vi "BRig_RT__Case_Exp__State_initTrial__LC_ENL__v10.vi"(6 "input_arrTrig":bool[](array[boolean]), 8 "input_dataTrial":u16[][](array[numeric]), 9 "input_dataExp":u16[](array[numeric]), 10 "input_dataLC":u16[](array[numeric]), 11 "input_dataCurrent":u16[](array[numeric])) -> (0 "output_dataTrial":u16[][](array[numeric]), 3 "output_dataCurrent":u16[](array[numeric]), 4 "output_arrTrig":bool[](array[boolean]))   [LabVIEW 2014]
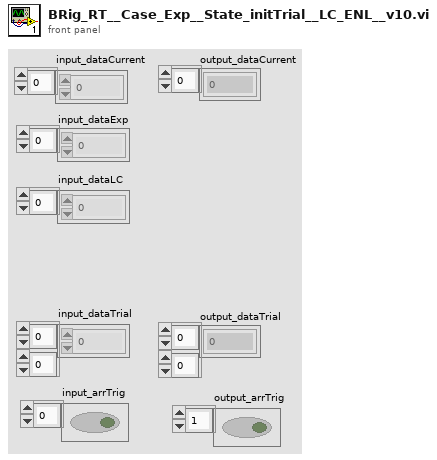
[diagram p1: front panel]
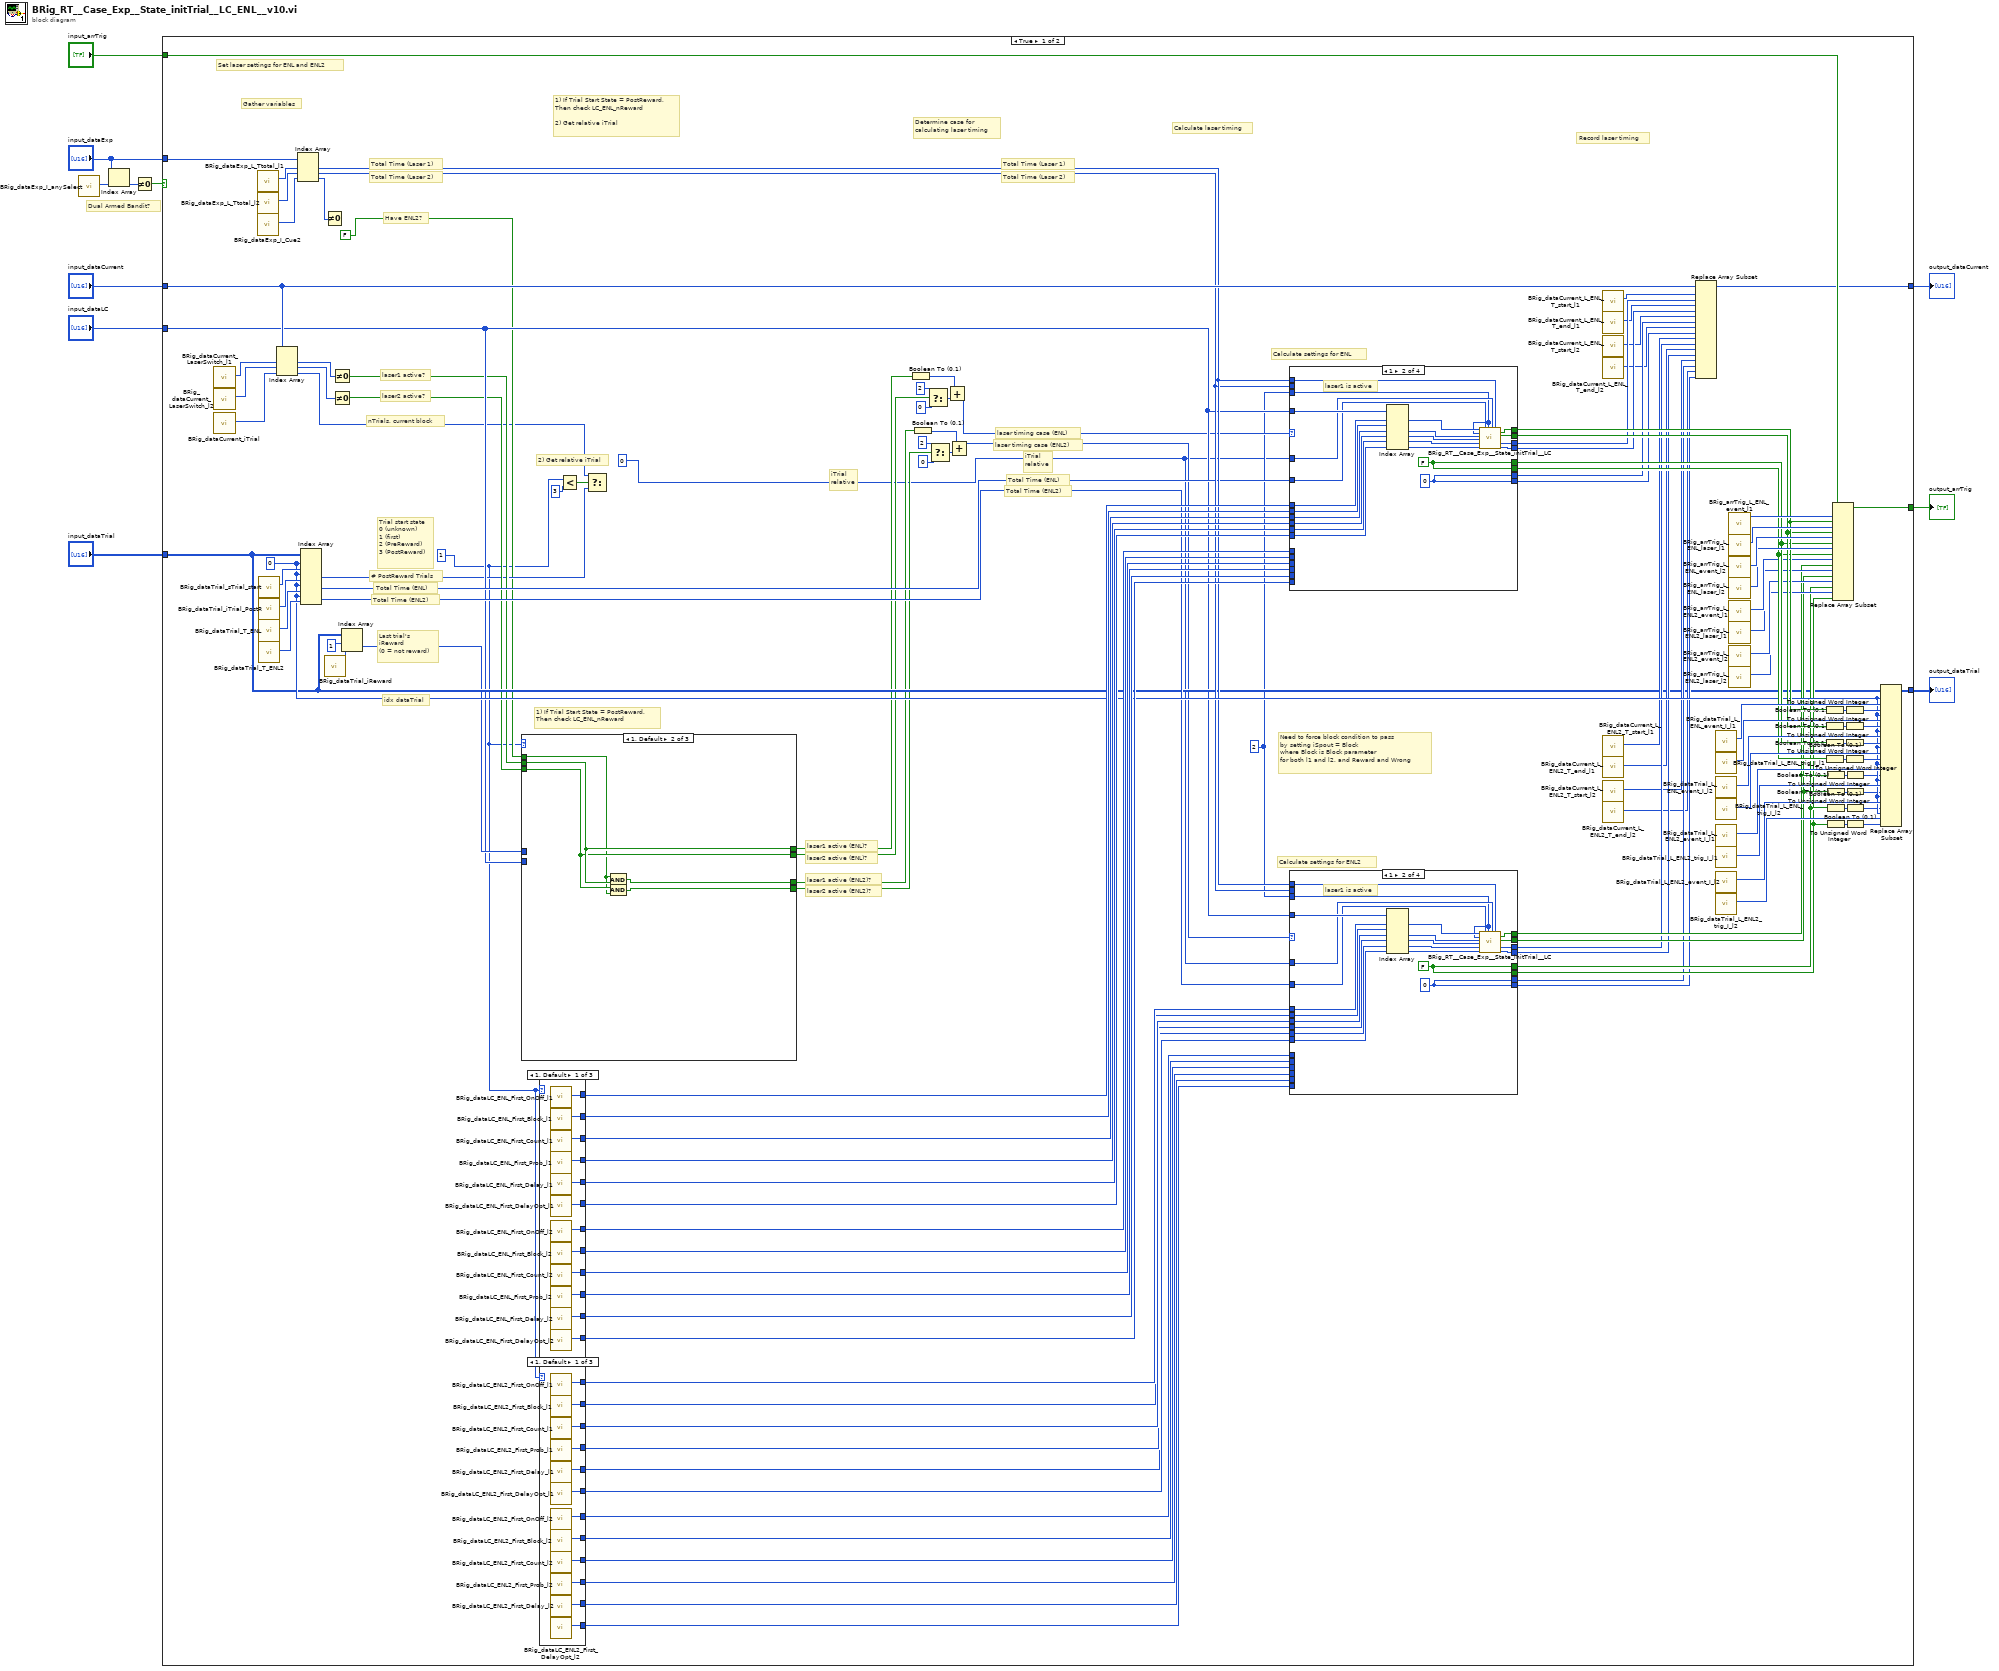
[diagram p0: block diagram]
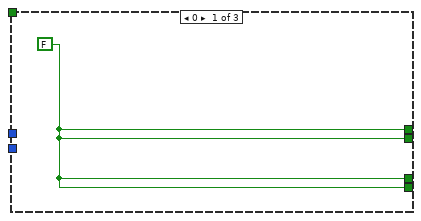
[diagram p2: hidden frame]
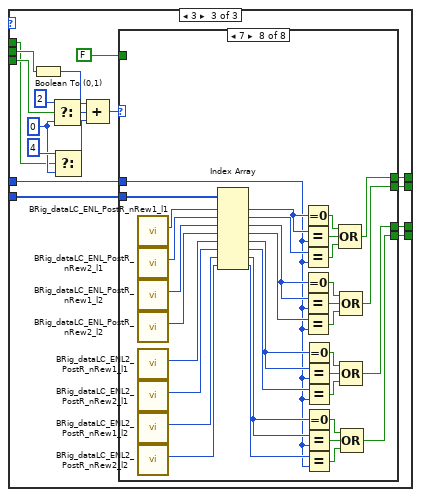
[diagram p3: hidden frame]
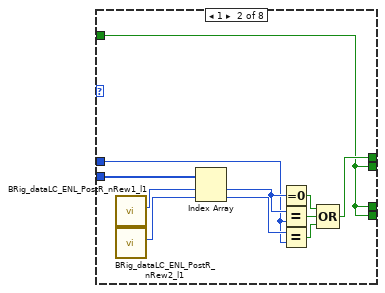
[diagram p5: hidden frame]
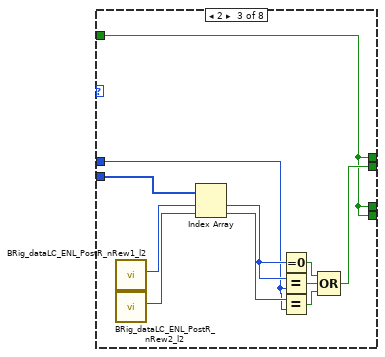
[diagram p6: hidden frame]
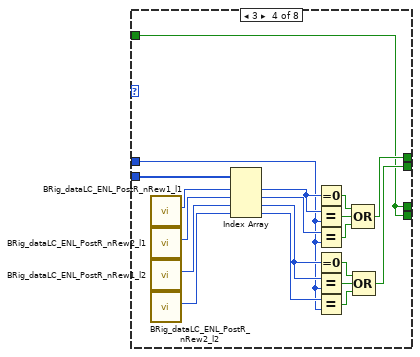
[diagram p7: hidden frame]
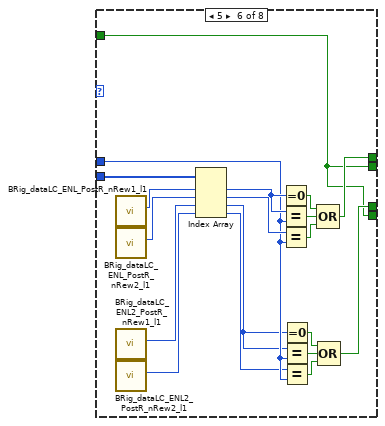
[diagram p9: hidden frame]
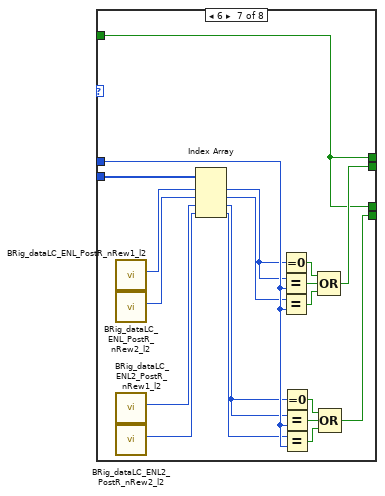
[diagram p10: hidden frame]
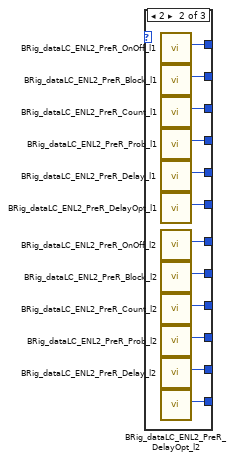
[diagram p11: hidden frame]
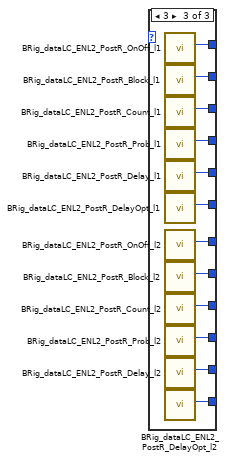
[diagram p12: hidden frame]
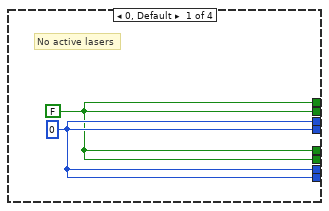
[diagram p13: hidden frame]
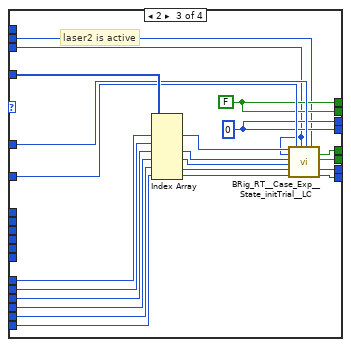
[diagram p14: hidden frame]
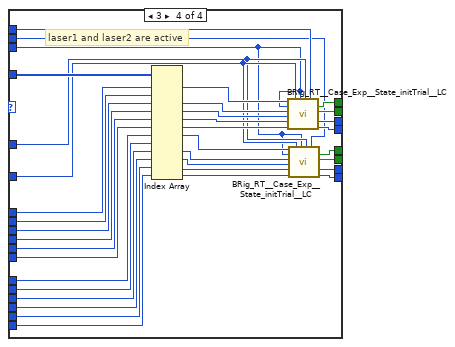
[diagram p15: hidden frame]
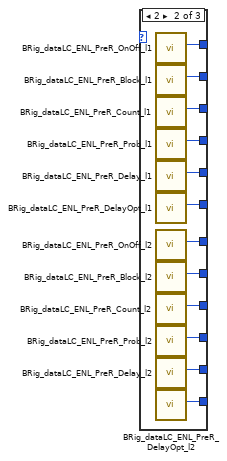
[diagram p16: hidden frame]
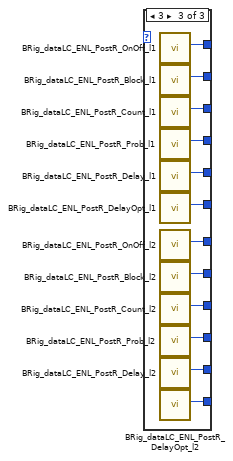
[diagram p17: hidden frame]
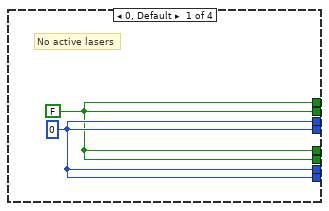
[diagram p18: hidden frame]
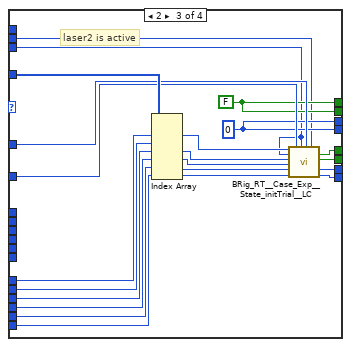
[diagram p19: hidden frame]
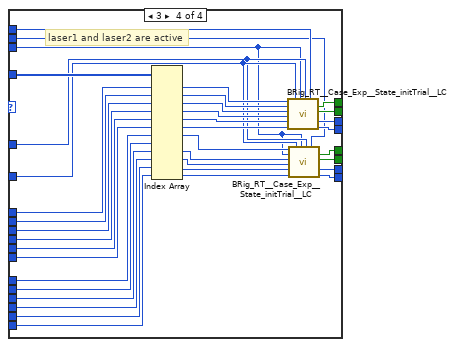
[diagram p20: hidden frame]
diagram:
  # "Dual Armed Bandit?"
  n1 = call "BRig_dataExp_I_anySelect.vi"() -> ("output_I_anySelect"=w4:i32)  [unwired: 11 in]
  n2 = Index Array(array="input_dataExp", index=w4) -> (element=w3:u16)
  n3 = Not Equal To 0?(x=w3) -> (x != 0?=w1:bool)
  n4 = case shown="True" w1 {
    tunnel: "input_arrTrig" -> [w135 w643]
    tunnel: [w134 w642] -> w10
    tunnel: [w113 w621] -> w9
    tunnel: "input_dataCurrent" -> [w112 w620]
    tunnel: [w111 w619] -> w7
    tunnel: "input_dataExp" -> [w88 w596]
    tunnel: "input_dataTrial" -> [w34 w541]
    tunnel: "input_dataLC" -> [w32 w539]
    frame True {
      w12 = u16 1
      w13 = u16 0
      w15 = u16 2 ("input_sState_start")
      w72 = 0
      # "Need to force block condition to pass\nby setting iSpout = Block\nwhere Block is Block parameter\nfor both l1 and l2, and Reward and Wrong"
      # "Record laser timing"
      # "Calculate laser timing"
      # "Total Time (ENL2)"
      # "Total Time (ENL)"
      # "iTrial\nrelative"
      # "Total Time (Laser 2)"
      # "Total Time (Laser 1)"
      # "laser timing case (ENL2)"
      # "Determine case for\ncalculating laser timing"
      # "2) Get relative iTrial"
      # "1) If Trial Start State = PostReward,\nThen check LC_ENL_nReward"
      # "laser2 active (ENL2)?"
      # "laser1 active (ENL2)?"
      # "laser2 active (ENL)?"
      # "laser1 active (ENL)?"
      # "1) If Trial Start State = PostReward,\nThen check LC_ENL_nReward\n\n2) Get relative iTrial"
      # "Gather variables"
      # "Last trial's\niReward\n(0 = not reward)"
      # "nTrials, current block"
      # "idx dataTrial"
      # "Total Time (ENL2)"
      # "Total Time (ENL)"
      # "# PostReward Trials"
      # "Have ENL2?"
      # "Total Time (Laser 2)"
      # "Total Time (Laser 1)"
      # "Calculate settings for ENL2"
      # "Calculate settings for ENL"
      # "Set laser settings for ENL and ENL2"
      # "iTrial\nrelative"
      # "laser timing case (ENL)"
      # "Trial start state\n0 (unknown)\n1 (first)\n2 (PreReward)\n3 (PostReward)"
      # "laser2 active?"
      # "laser1 active?"
      n5 = call "BRig_dataCurrent_LaserSwitch_l1.vi"() -> ("output_LaserSwitch_l1"=w144:i32)  [unwired: 11 in]
      n6 = call "BRig_dataCurrent_LaserSwitch_l2.vi"() -> ("output_LaserSwitch_l2"=w143:i32)  [unwired: 11 in]
      n7 = call "BRig_dataCurrent_iTrial.vi"() -> ("output_iTrial"=w85:i32)  [unwired: 11 in]
      n8 = call "BRig_dataExp_L_Ttotal_l1.vi"() -> ("output_L_Ttotal_l1"=w89:i32)  [unwired: 11 in]
      n9 = call "BRig_dataExp_L_Ttotal_l2.vi"() -> ("output_L_Ttotal_l2"=w90:i32)  [unwired: 11 in]
      n10 = call "BRig_dataExp_I_Cue2.vi"() -> ("output_I_Cue2"=w40:i32)  [unwired: 11 in]
      n11 = call "BRig_dataTrial_sTrial_start.vi"() -> ("output_sTrial_start"=w140:i32)  [unwired: 11 in]
      n12 = call "BRig_dataTrial_iTrial_PostR.vi"() -> ("output_iTrial_PostR"=w86:i32)  [unwired: 11 in]
      n13 = call "BRig_dataTrial_T_ENL.vi"() -> ("output_T_ENL"=w87:i32)  [unwired: 11 in]
      n14 = call "BRig_dataTrial_T_ENL2.vi"() -> ("output_T_ENL2"=w84:i32)  [unwired: 11 in]
      n15 = Index Array(array=w112, index #1=w144, index #2=w143, index #3=w85) -> (element #1=w142:u16, element #2=w141:u16, element #3=w14:u16)
      n16 = Index Array(array=w88, index #1=w89, index #2=w90, index #3=w40) -> (element #1=w66:u16, element #2=w65:u16, element #3=w39:u16)
      n17 = Index Array(array=w34, index (row) #1=w72, index (col) #1=w140, index (row) #2=w72, index (col) #2=w86, index (row) #3=w72, index (col) #3=w87, index (row) #4=w72, index (col) #4=w84) -> (element #2=w27:u16, element #3=w38:u16, element #4=w37:u16)  [unwired: 1 out]
      n18 = Not Equal To 0?(x=w39) -> ()  [unwired: 1 out]
      n19 = call "BRig_dataTrial_iReward.vi"() -> ("output_iReward"=w35:i32)  [unwired: 11 in]
      n20 = Not Equal To 0?(x=w142) -> (x != 0?=w30:bool)
      n21 = Not Equal To 0?(x=w141) -> (x != 0?=w31:bool)
      n22 = Index Array(array=w34, index (row)=1 ("disabled index (row)"), index (col)=w35) -> (element=w33:u16)
      n23 = case shown="1, Default" w12 {
        tunnel: w33 -> [_ _ w159]
        tunnel: w32 -> [_ _ w160]
        tunnel: w31 -> [_ w149 w152]
        tunnel: w30 -> [_ w150 w153]
        tunnel: FALSE -> [_ w148 w151]
        tunnel: [w145 w150 w158] -> w26
        tunnel: [w145 w149 w157] -> w25
        tunnel: [w145 w147 w156] -> w20
        tunnel: [w145 w146 w155] -> w19
        frame 0 {
          w145 = FALSE
        }
        frame 1, Default {
          n24 = And(x=w148, y=w150) -> (x .and. y?=w147:bool)
          n25 = And(x=w149, y=w148) -> (x .and. y?=w146:bool)
        }
        frame 3 {
          w165 = i16 0 ("f")
          n26 = Boolean To (0,1)(Boolean=w153) -> (0, 1=w163:i16)
          n27 = Select(t=i16 2, s=w152, f=w165) -> (s? t:f=w164:i16)
          n28 = Select(t=i16 4, s=w151, f=w165) -> (s? t:f=w162:i16)
          n29 = Compound Arithmetic op=ADD(w163, w164, w162) -> (w161:i16)
          n30 = case shown="7" w161 {
            tunnel: w160 -> [_ w172 w183 w195 _ w222 w245 w268]
            tunnel: w159 -> [_ w171 w182 w194 _ w218 w241 w253]
            tunnel: [w168 w170 w180 w193 w210 w217 w238 w252] -> w158
            tunnel: [w168 w169 w181 w192 w210 w215 w240 w251] -> w157
            tunnel: [w168 w169 w180 w191 w210 w216 w238 w250] -> w156
            tunnel: [w168 w169 w180 w191 w210 w215 w239 w249] -> w155
            tunnel: FALSE -> [w168 w169 w180 w191 w210 w215 w238 _]
            frame 0, Default {
            }
            frame 1 {
              n31 = call "BRig_dataLC_ENL_PostR_nRew1_l1.vi"() -> ("output_ENL_PostR_nRew1_l1"=w179:i32)  [unwired: 11 in]
              n32 = call "BRig_dataLC_ENL_PostR_nRew2_l1.vi"() -> ("output_ENL_PostR_nRew2_l1"=w178:i32)  [unwired: 11 in]
              n33 = Index Array(array=w172, index #1=w179, index #2=w178) -> (element #1=w174:u16, element #2=w173:u16)
              n34 = Equal To 0?(x=w174) -> (x = 0?=w175:bool)
              n35 = Equal?(x=w174, y=w171) -> (x = y?=w176:bool)
              n36 = Equal?(x=w173, y=w171) -> (x = y?=w177:bool)
              n37 = Compound Arithmetic op=OR(w175, w176, w177) -> (w170:bool)
            }
            frame 2 {
              n38 = call "BRig_dataLC_ENL_PostR_nRew1_l2.vi"() -> ("output_ENL_PostR_nRew1_l2"=w190:i32)  [unwired: 11 in]
              n39 = call "BRig_dataLC_ENL_PostR_nRew2_l2.vi"() -> ("output_ENL_PostR_nRew2_l2"=w189:i32)  [unwired: 11 in]
              n40 = Index Array(array=w183, index #1=w190, index #2=w189) -> (element #1=w184:u16, element #2=w185:u16)
              n41 = Equal To 0?(x=w184) -> (x = 0?=w187:bool)
              n42 = Equal?(x=w184, y=w182) -> (x = y?=w186:bool)
              n43 = Equal?(x=w185, y=w182) -> (x = y?=w188:bool)
              n44 = Compound Arithmetic op=OR(w187, w186, w188) -> (w181:bool)
            }
            frame 3 {
              n45 = call "BRig_dataLC_ENL_PostR_nRew1_l1.vi"() -> ("output_ENL_PostR_nRew1_l1"=w209:i32)  [unwired: 11 in]
              n46 = call "BRig_dataLC_ENL_PostR_nRew2_l1.vi"() -> ("output_ENL_PostR_nRew2_l1"=w208:i32)  [unwired: 11 in]
              n47 = call "BRig_dataLC_ENL_PostR_nRew1_l2.vi"() -> ("output_ENL_PostR_nRew1_l2"=w207:i32)  [unwired: 11 in]
              n48 = call "BRig_dataLC_ENL_PostR_nRew2_l2.vi"() -> ("output_ENL_PostR_nRew2_l2"=w206:i32)  [unwired: 11 in]
              n49 = Index Array(array=w195, index #1=w209, index #2=w208, index #3=w207, index #4=w206) -> (element #1=w199:u16, element #2=w198:u16, element #3=w196:u16, element #4=w197:u16)
              n50 = Equal To 0?(x=w199) -> (x = 0?=w200:bool)
              n51 = Equal?(x=w199, y=w194) -> (x = y?=w201:bool)
              n52 = Equal?(x=w198, y=w194) -> (x = y?=w202:bool)
              n53 = Equal To 0?(x=w196) -> (x = 0?=w204:bool)
              n54 = Equal?(x=w196, y=w194) -> (x = y?=w203:bool)
              n55 = Equal?(x=w197, y=w194) -> (x = y?=w205:bool)
              n56 = Compound Arithmetic op=OR(w200, w201, w202) -> (w193:bool)
              n57 = Compound Arithmetic op=OR(w204, w203, w205) -> (w192:bool)
            }
            frame 4 {
            }
            frame 5 {
              n58 = call "BRig_dataLC_ENL_PostR_nRew1_l1.vi"() -> ("output_ENL_PostR_nRew1_l1"=w229:i32)  [unwired: 11 in]
              n59 = call "BRig_dataLC_ENL_PostR_nRew2_l1.vi"() -> ("output_ENL_PostR_nRew2_l1"=w228:i32)  [unwired: 11 in]
              n60 = call "BRig_dataLC_ENL2_PostR_nRew1_l1.vi"() -> ("output_ENL2_PostR_nRew1_l1"=w214:i32)  [unwired: 11 in]
              n61 = call "BRig_dataLC_ENL2_PostR_nRew2_l1.vi"() -> ("output_ENL2_PostR_nRew2_l1"=w213:i32)  [unwired: 11 in]
              n62 = Index Array(array=w222, index #1=w229, index #2=w228, index #3=w214, index #4=w213) -> (element #1=w224:u16, element #2=w223:u16, element #3=w212:u16, element #4=w211:u16)
              n63 = Equal To 0?(x=w224) -> (x = 0?=w225:bool)
              n64 = Equal?(x=w224, y=w218) -> (x = y?=w226:bool)
              n65 = Equal?(x=w223, y=w218) -> (x = y?=w227:bool)
              n66 = Equal To 0?(x=w212) -> (x = 0?=w221:bool)
              n67 = Equal?(x=w212, y=w218) -> (x = y?=w220:bool)
              n68 = Equal?(x=w211, y=w218) -> (x = y?=w219:bool)
              n69 = Compound Arithmetic op=OR(w225, w226, w227) -> (w217:bool)
              n70 = Compound Arithmetic op=OR(w221, w220, w219) -> (w216:bool)
            }
            frame 6 {
              n71 = call "BRig_dataLC_ENL_PostR_nRew1_l2.vi"() -> ("output_ENL_PostR_nRew1_l2"=w237:i32)  [unwired: 11 in]
              n72 = call "BRig_dataLC_ENL_PostR_nRew2_l2.vi"() -> ("output_ENL_PostR_nRew2_l2"=w236:i32)  [unwired: 11 in]
              n73 = call "BRig_dataLC_ENL2_PostR_nRew1_l2.vi"() -> ("output_ENL2_PostR_nRew1_l2"=w233:i32)  [unwired: 11 in]
              n74 = call "BRig_dataLC_ENL2_PostR_nRew2_l2.vi"() -> ("output_ENL2_PostR_nRew2_l2"=w232:i32)  [unwired: 11 in]
              n75 = Index Array(array=w245, index #1=w237, index #2=w236, index #3=w233, index #4=w232) -> (element #1=w235:u16, element #2=w234:u16, element #3=w231:u16, element #4=w230:u16)
              n76 = Equal To 0?(x=w235) -> (x = 0?=w247:bool)
              n77 = Equal?(x=w235, y=w241) -> (x = y?=w246:bool)
              n78 = Equal?(x=w234, y=w241) -> (x = y?=w248:bool)
              n79 = Equal To 0?(x=w231) -> (x = 0?=w243:bool)
              n80 = Equal?(x=w231, y=w241) -> (x = y?=w244:bool)
              n81 = Equal?(x=w230, y=w241) -> (x = y?=w242:bool)
              n82 = Compound Arithmetic op=OR(w247, w246, w248) -> (w240:bool)
              n83 = Compound Arithmetic op=OR(w243, w244, w242) -> (w239:bool)
            }
            frame 7 {
              n84 = call "BRig_dataLC_ENL_PostR_nRew1_l1.vi"() -> ("output_ENL_PostR_nRew1_l1"=w282:i32)  [unwired: 11 in]
              n85 = call "BRig_dataLC_ENL_PostR_nRew2_l1.vi"() -> ("output_ENL_PostR_nRew2_l1"=w281:i32)  [unwired: 11 in]
              n86 = call "BRig_dataLC_ENL_PostR_nRew1_l2.vi"() -> ("output_ENL_PostR_nRew1_l2"=w280:i32)  [unwired: 11 in]
              n87 = call "BRig_dataLC_ENL_PostR_nRew2_l2.vi"() -> ("output_ENL_PostR_nRew2_l2"=w279:i32)  [unwired: 11 in]
              n88 = call "BRig_dataLC_ENL2_PostR_nRew1_l1.vi"() -> ("output_ENL2_PostR_nRew1_l1"=w267:i32)  [unwired: 11 in]
              n89 = call "BRig_dataLC_ENL2_PostR_nRew2_l1.vi"() -> ("output_ENL2_PostR_nRew2_l1"=w266:i32)  [unwired: 11 in]
              n90 = call "BRig_dataLC_ENL2_PostR_nRew1_l2.vi"() -> ("output_ENL2_PostR_nRew1_l2"=w265:i32)  [unwired: 11 in]
              n91 = call "BRig_dataLC_ENL2_PostR_nRew2_l2.vi"() -> ("output_ENL2_PostR_nRew2_l2"=w264:i32)  [unwired: 11 in]
              n92 = Index Array(array=w268, index #1=w282, index #2=w281, index #3=w280, index #4=w279, index #5=w267, index #6=w266, index #7=w265, index #8=w264) -> (element #1=w272:u16, element #2=w271:u16, element #3=w269:u16, element #4=w270:u16, element #5=w257:u16, element #6=w256:u16, element #7=w254:u16, element #8=w255:u16)
              n93 = Equal To 0?(x=w272) -> (x = 0?=w273:bool)
              n94 = Equal?(x=w272, y=w253) -> (x = y?=w274:bool)
              n95 = Equal?(x=w271, y=w253) -> (x = y?=w275:bool)
              n96 = Equal To 0?(x=w269) -> (x = 0?=w277:bool)
              n97 = Equal?(x=w269, y=w253) -> (x = y?=w276:bool)
              n98 = Equal?(x=w270, y=w253) -> (x = y?=w278:bool)
              n99 = Equal To 0?(x=w257) -> (x = 0?=w263:bool)
              n100 = Equal?(x=w257, y=w253) -> (x = y?=w262:bool)
              n101 = Equal?(x=w256, y=w253) -> (x = y?=w261:bool)
              n102 = Equal To 0?(x=w254) -> (x = 0?=w259:bool)
              n103 = Equal?(x=w254, y=w253) -> (x = y?=w260:bool)
              n104 = Equal?(x=w255, y=w253) -> (x = y?=w258:bool)
              n105 = Compound Arithmetic op=OR(w273, w274, w275) -> (w252:bool)
              n106 = Compound Arithmetic op=OR(w277, w276, w278) -> (w251:bool)
              n107 = Compound Arithmetic op=OR(w263, w262, w261) -> (w250:bool)
              n108 = Compound Arithmetic op=OR(w259, w260, w258) -> (w249:bool)
            }
          }
        }
      }
      n109 = case shown="1, Default" w12 {
        tunnel: [w412 w424 w436] -> w102
        tunnel: [w411 w423 w425] -> w101
        tunnel: [w410 w422 w426] -> w100
        tunnel: [w409 w421 w427] -> w99
        tunnel: [w408 w420 w428] -> w98
        tunnel: [w407 w419 w429] -> w97
        tunnel: [w406 w418 w435] -> w96
        tunnel: [w405 w417 w434] -> w95
        tunnel: [w404 w416 w433] -> w94
        tunnel: [w403 w415 w432] -> w93
        tunnel: [w402 w414 w431] -> w92
        tunnel: [w401 w413 w430] -> w91
        frame 1, Default {
          n110 = call "BRig_dataLC_ENL_First_OnOff_l1.vi"() -> ("output_ENL_First_OnOff"=w412:i32)  [unwired: 11 in]
          n111 = call "BRig_dataLC_ENL_First_Block_l1.vi"() -> ("output_ENL_First_Block"=w411:i32)  [unwired: 11 in]
          n112 = call "BRig_dataLC_ENL_First_Count_l1.vi"() -> ("output_ENL_First_Count"=w410:i32)  [unwired: 11 in]
          n113 = call "BRig_dataLC_ENL_First_Prob_l1.vi"() -> ("output_ENL_First_Prob"=w409:i32)  [unwired: 11 in]
          n114 = call "BRig_dataLC_ENL_First_Delay_l1.vi"() -> ("output_ENL_First_Delay"=w408:i32)  [unwired: 11 in]
          n115 = call "BRig_dataLC_ENL_First_DelayOpt_l1.vi"() -> ("output_ENL_First_DelayOpt"=w407:i32)  [unwired: 11 in]
          n116 = call "BRig_dataLC_ENL_First_OnOff_l2.vi"() -> ("output_ENL_First_OnOff_l2"=w406:i32)  [unwired: 11 in]
          n117 = call "BRig_dataLC_ENL_First_Block_l2.vi"() -> ("output_ENL_First_Block_l2"=w405:i32)  [unwired: 11 in]
          n118 = call "BRig_dataLC_ENL_First_Count_l2.vi"() -> ("output_ENL_First_Count_l2"=w404:i32)  [unwired: 11 in]
          n119 = call "BRig_dataLC_ENL_First_Prob_l2.vi"() -> ("output_ENL_First_Prob_l2"=w403:i32)  [unwired: 11 in]
          n120 = call "BRig_dataLC_ENL_First_Delay_l2.vi"() -> ("output_ENL_First_Delay_l2"=w402:i32)  [unwired: 11 in]
          n121 = call "BRig_dataLC_ENL_First_DelayOpt_l2.vi"() -> ("output_ENL_First_DelayOpt_l2"=w401:i32)  [unwired: 11 in]
        }
        frame 2 {
          n122 = call "BRig_dataLC_ENL_PreR_OnOff_l1.vi"() -> ("output_ENL_PreR_OnOff"=w424:i32)  [unwired: 11 in]
          n123 = call "BRig_dataLC_ENL_PreR_Block_l1.vi"() -> ("output_ENL_PreR_Block"=w423:i32)  [unwired: 11 in]
          n124 = call "BRig_dataLC_ENL_PreR_Count_l1.vi"() -> ("output_ENL_PreR_Count"=w422:i32)  [unwired: 11 in]
          n125 = call "BRig_dataLC_ENL_PreR_Prob_l1.vi"() -> ("output_ENL_PreR_Prob"=w421:i32)  [unwired: 11 in]
          n126 = call "BRig_dataLC_ENL_PreR_Delay_l1.vi"() -> ("output_ENL_PreR_Delay"=w420:i32)  [unwired: 11 in]
          n127 = call "BRig_dataLC_ENL_PreR_DelayOpt_l1.vi"() -> ("output_ENL_PreR_DelayOpt"=w419:i32)  [unwired: 11 in]
          n128 = call "BRig_dataLC_ENL_PreR_OnOff_l2.vi"() -> ("output_ENL_PreR_OnOff_l2"=w418:i32)  [unwired: 11 in]
          n129 = call "BRig_dataLC_ENL_PreR_Block_l2.vi"() -> ("output_ENL_PreR_Block_l2"=w417:i32)  [unwired: 11 in]
          n130 = call "BRig_dataLC_ENL_PreR_Count_l2.vi"() -> ("output_ENL_PreR_Count_l2"=w416:i32)  [unwired: 11 in]
          n131 = call "BRig_dataLC_ENL_PreR_Prob_l2.vi"() -> ("output_ENL_PreR_Prob_l2"=w415:i32)  [unwired: 11 in]
          n132 = call "BRig_dataLC_ENL_PreR_Delay_l2.vi"() -> ("output_ENL_PreR_Delay_l2"=w414:i32)  [unwired: 11 in]
          n133 = call "BRig_dataLC_ENL_PreR_DelayOpt_l2.vi"() -> ("output_ENL_PreR_DelayOpt_l2"=w413:i32)  [unwired: 11 in]
        }
        frame 3 {
          n134 = call "BRig_dataLC_ENL_PostR_OnOff_l1.vi"() -> ("output_ENL_PostR_OnOff"=w436:i32)  [unwired: 11 in]
          n135 = call "BRig_dataLC_ENL_PostR_Block_l1.vi"() -> ("output_ENL_PostR_Block"=w425:i32)  [unwired: 11 in]
          n136 = call "BRig_dataLC_ENL_PostR_Count_l1.vi"() -> ("output_ENL_PostR_Count"=w426:i32)  [unwired: 11 in]
          n137 = call "BRig_dataLC_ENL_PostR_Prob_l1.vi"() -> ("output_ENL_PostR_Prob"=w427:i32)  [unwired: 11 in]
          n138 = call "BRig_dataLC_ENL_PostR_Delay_l1.vi"() -> ("output_ENL_PostR_Delay"=w428:i32)  [unwired: 11 in]
          n139 = call "BRig_dataLC_ENL_PostR_DelayOpt_l1.vi"() -> ("output_ENL_PostR_DelayOpt"=w429:i32)  [unwired: 11 in]
          n140 = call "BRig_dataLC_ENL_PostR_OnOff_l2.vi"() -> ("output_ENL_PostR_OnOff_l2"=w435:i32)  [unwired: 11 in]
          n141 = call "BRig_dataLC_ENL_PostR_Block_l2.vi"() -> ("output_ENL_PostR_Block_l2"=w434:i32)  [unwired: 11 in]
          n142 = call "BRig_dataLC_ENL_PostR_Count_l2.vi"() -> ("output_ENL_PostR_Count_l2"=w433:i32)  [unwired: 11 in]
          n143 = call "BRig_dataLC_ENL_PostR_Prob_l2.vi"() -> ("output_ENL_PostR_Prob_l2"=w432:i32)  [unwired: 11 in]
          n144 = call "BRig_dataLC_ENL_PostR_Delay_l2.vi"() -> ("output_ENL_PostR_Delay_l2"=w431:i32)  [unwired: 11 in]
          n145 = call "BRig_dataLC_ENL_PostR_DelayOpt_l2.vi"() -> ("output_ENL_PostR_DelayOpt_l2"=w430:i32)  [unwired: 11 in]
        }
      }
      n146 = case shown="1, Default" w12 {
        tunnel: [w294 w306 w318] -> w64
        tunnel: [w293 w305 w317] -> w63
        tunnel: [w292 w304 w316] -> w62
        tunnel: [w291 w303 w315] -> w61
        tunnel: [w290 w302 w314] -> w60
        tunnel: [w289 w301 w313] -> w59
        tunnel: [w288 w300 w312] -> w58
        tunnel: [w287 w299 w311] -> w57
        tunnel: [w286 w298 w310] -> w56
        tunnel: [w285 w297 w309] -> w55
        tunnel: [w284 w296 w308] -> w54
        tunnel: [w283 w295 w307] -> w53
        frame 1, Default {
          n147 = call "BRig_dataLC_ENL2_First_OnOff_l1.vi"() -> ("output_ENL2_First_OnOff"=w294:i32)  [unwired: 11 in]
          n148 = call "BRig_dataLC_ENL2_First_Block_l1.vi"() -> ("output_ENL2_First_Block"=w293:i32)  [unwired: 11 in]
          n149 = call "BRig_dataLC_ENL2_First_Count_l1.vi"() -> ("output_ENL2_First_Count"=w292:i32)  [unwired: 11 in]
          n150 = call "BRig_dataLC_ENL2_First_Prob_l1.vi"() -> ("output_ENL2_First_Prob"=w291:i32)  [unwired: 11 in]
          n151 = call "BRig_dataLC_ENL2_First_Delay_l1.vi"() -> ("output_ENL2_First_Delay"=w290:i32)  [unwired: 11 in]
          n152 = call "BRig_dataLC_ENL2_First_DelayOpt_l1.vi"() -> ("output_ENL2_First_DelayOpt"=w289:i32)  [unwired: 11 in]
          n153 = call "BRig_dataLC_ENL2_First_OnOff_l2.vi"() -> ("output_ENL2_First_OnOff_l2"=w288:i32)  [unwired: 11 in]
          n154 = call "BRig_dataLC_ENL2_First_Block_l2.vi"() -> ("output_ENL2_First_Block_l2"=w287:i32)  [unwired: 11 in]
          n155 = call "BRig_dataLC_ENL2_First_Count_l2.vi"() -> ("output_ENL2_First_Count_l2"=w286:i32)  [unwired: 11 in]
          n156 = call "BRig_dataLC_ENL2_First_Prob_l2.vi"() -> ("output_ENL2_First_Prob_l2"=w285:i32)  [unwired: 11 in]
          n157 = call "BRig_dataLC_ENL2_First_Delay_l2.vi"() -> ("output_ENL2_First_Delay_l2"=w284:i32)  [unwired: 11 in]
          n158 = call "BRig_dataLC_ENL2_First_DelayOpt_l2.vi"() -> ("output_ENL2_First_DelayOpt_l2"=w283:i32)  [unwired: 11 in]
        }
        frame 2 {
          n159 = call "BRig_dataLC_ENL2_PreR_OnOff_l1.vi"() -> ("output_ENL2_PreR_OnOff"=w306:i32)  [unwired: 11 in]
          n160 = call "BRig_dataLC_ENL2_PreR_Block_l1.vi"() -> ("output_ENL2_PreR_Block"=w305:i32)  [unwired: 11 in]
          n161 = call "BRig_dataLC_ENL2_PreR_Count_l1.vi"() -> ("output_ENL2_PreR_Count"=w304:i32)  [unwired: 11 in]
          n162 = call "BRig_dataLC_ENL2_PreR_Prob_l1.vi"() -> ("output_ENL2_PreR_Prob"=w303:i32)  [unwired: 11 in]
          n163 = call "BRig_dataLC_ENL2_PreR_Delay_l1.vi"() -> ("output_ENL2_PreR_Delay"=w302:i32)  [unwired: 11 in]
          n164 = call "BRig_dataLC_ENL2_PreR_DelayOpt_l1.vi"() -> ("output_ENL2_PreR_DelayOpt"=w301:i32)  [unwired: 11 in]
          n165 = call "BRig_dataLC_ENL2_PreR_OnOff_l2.vi"() -> ("output_ENL2_PreR_OnOff_l2"=w300:i32)  [unwired: 11 in]
          n166 = call "BRig_dataLC_ENL2_PreR_Block_l2.vi"() -> ("output_ENL2_PreR_Block_l2"=w299:i32)  [unwired: 11 in]
          n167 = call "BRig_dataLC_ENL2_PreR_Count_l2.vi"() -> ("output_ENL2_PreR_Count_l2"=w298:i32)  [unwired: 11 in]
          n168 = call "BRig_dataLC_ENL2_PreR_Prob_l2.vi"() -> ("output_ENL2_PreR_Prob_l2"=w297:i32)  [unwired: 11 in]
          n169 = call "BRig_dataLC_ENL2_PreR_Delay_l2.vi"() -> ("output_ENL2_PreR_Delay_l2"=w296:i32)  [unwired: 11 in]
          n170 = call "BRig_dataLC_ENL2_PreR_DelayOpt_l2.vi"() -> ("output_ENL2_PreR_DelayOpt_l2"=w295:i32)  [unwired: 11 in]
        }
        frame 3 {
          n171 = call "BRig_dataLC_ENL2_PostR_OnOff_l1.vi"() -> ("output_ENL2_PostR_OnOff"=w318:i32)  [unwired: 11 in]
          n172 = call "BRig_dataLC_ENL2_PostR_Block_l1.vi"() -> ("output_ENL2_PostR_Block"=w317:i32)  [unwired: 11 in]
          n173 = call "BRig_dataLC_ENL2_PostR_Count_l1.vi"() -> ("output_ENL2_PostR_Count"=w316:i32)  [unwired: 11 in]
          n174 = call "BRig_dataLC_ENL2_PostR_Prob_l1.vi"() -> ("output_ENL2_PostR_Prob"=w315:i32)  [unwired: 11 in]
          n175 = call "BRig_dataLC_ENL2_PostR_Delay_l1.vi"() -> ("output_ENL2_PostR_Delay"=w314:i32)  [unwired: 11 in]
          n176 = call "BRig_dataLC_ENL2_PostR_DelayOpt_l1.vi"() -> ("output_ENL2_PostR_DelayOpt"=w313:i32)  [unwired: 11 in]
          n177 = call "BRig_dataLC_ENL2_PostR_OnOff_l2.vi"() -> ("output_ENL2_PostR_OnOff_l2"=w312:i32)  [unwired: 11 in]
          n178 = call "BRig_dataLC_ENL2_PostR_Block_l2.vi"() -> ("output_ENL2_PostR_Block_l2"=w311:i32)  [unwired: 11 in]
          n179 = call "BRig_dataLC_ENL2_PostR_Count_l2.vi"() -> ("output_ENL2_PostR_Count_l2"=w310:i32)  [unwired: 11 in]
          n180 = call "BRig_dataLC_ENL2_PostR_Prob_l2.vi"() -> ("output_ENL2_PostR_Prob_l2"=w309:i32)  [unwired: 11 in]
          n181 = call "BRig_dataLC_ENL2_PostR_Delay_l2.vi"() -> ("output_ENL2_PostR_Delay_l2"=w308:i32)  [unwired: 11 in]
          n182 = call "BRig_dataLC_ENL2_PostR_DelayOpt_l2.vi"() -> ("output_ENL2_PostR_DelayOpt_l2"=w307:i32)  [unwired: 11 in]
        }
      }
      n183 = Less?(x=w12, y=u16 3) -> (x < y?=w28:bool)
      n184 = Select(t=w14, s=w28, f=w27) -> ()  [unwired: 1 out]
      n185 = Boolean To (0,1)(Boolean=w26) -> (0, 1=w137:i16)
      n186 = Boolean To (0,1)(Boolean=w20) -> (0, 1=w23:i16)
      n187 = Select(t=i16 2, s=w25, f=i16 0) -> (s? t:f=w138:i16)
      n188 = Select(t=i16 2, s=w19, f=i16 0) -> (s? t:f=w22:i16)
      n189 = Add(x=w137, y=w138) -> (x+y=w18:i16)
      n190 = Add(x=w23, y=w22) -> (x+y=w17:i16)
      n191 = case shown="1" w18 {
        tunnel: w32 -> [_ w460 w482 w519]
        tunnel: w15 -> [_ w439 w461 w483]
        tunnel: w38 -> [_ w454 w476 w507]
        tunnel: w13 -> [_ w453 w475 w506]
        tunnel: [w437 w452 w464 w505] -> w124
        tunnel: [w437 w451 w464 w504] -> w118
        tunnel: [w438 w450 w463 w503] -> w109
        tunnel: [w438 w449 w463 w502] -> w107
        tunnel: [w437 w442 w474 w501] -> w114
        tunnel: [w438 w441 w473 w500] -> w105
        tunnel: [w437 w442 w472 w499] -> w116
        tunnel: [w438 w441 w471 w498] -> w103
        tunnel: w102 -> [_ w448 _ w497]
        tunnel: w101 -> [_ w447 _ w496]
        tunnel: w100 -> [_ w446 _ w495]
        tunnel: w99 -> [_ w445 _ w494]
        tunnel: w98 -> [_ w444 _ w493]
        tunnel: w97 -> [_ w443 _ w492]
        tunnel: w96 -> [_ _ w470 w491]
        tunnel: w95 -> [_ _ w469 w490]
        tunnel: w94 -> [_ _ w468 w489]
        tunnel: w93 -> [_ _ w467 w488]
        tunnel: w92 -> [_ _ w466 w487]
        tunnel: w91 -> [_ _ w465 w486]
        tunnel: w66 -> [_ w440 _ w485]
        tunnel: w65 -> [_ _ w462 w484]
        frame 0, Default {
          w438 = u16 0
          w437 = FALSE
          # "No active lasers"
        }
        frame 1 {
          w441 = u16 0
          w442 = FALSE
          # "laser1 is active"
          n192 = Index Array(array=w460, index #1=w448, index #2=w447, index #3=w446, index #4=w445, index #5=w444, index #6=w443) -> (element #1=w459:u16, element #3=w458:u16, element #4=w457:u16, element #5=w456:u16, element #6=w455:u16)  [unwired: 1 out]
          n193 = call "BRig_RT__Case_Exp__State_initTrial__LC.vi"("input_L_OnOff"=w459, "input_L_Block"=w439, "input_L_Count"=w458, "input_L_Prob"=w457, "input_L_Tdelay"=w456, "input_L_delayOpt"=w455, "input_T_state"=w454, "input_iSpout"=w439, "input_iTrial_relative"=w453, "input_L_T"=w440) -> ("output_LC_Event"=w452:bool, "output_LC_Laser"=w451:bool, "output_L_Tstart"=w450:u16, "output_L_Tend"=w449:u16)  [unwired: 6 in]
        }
        frame 2 {
          w463 = u16 0
          w464 = FALSE
          # "laser2 is active"
          n194 = Index Array(array=w482, index #1=w470, index #2=w469, index #3=w468, index #4=w467, index #5=w466, index #6=w465) -> (element #1=w477:u16, element #3=w478:u16, element #4=w479:u16, element #5=w480:u16, element #6=w481:u16)  [unwired: 1 out]
          n195 = call "BRig_RT__Case_Exp__State_initTrial__LC.vi"("input_L_OnOff"=w477, "input_L_Block"=w461, "input_L_Count"=w478, "input_L_Prob"=w479, "input_L_Tdelay"=w480, "input_L_delayOpt"=w481, "input_T_state"=w476, "input_iSpout"=w461, "input_iTrial_relative"=w475, "input_L_T"=w462) -> ("output_LC_Event"=w472:bool, "output_LC_Laser"=w474:bool, "output_L_Tstart"=w473:u16, "output_L_Tend"=w471:u16)  [unwired: 6 in]
        }
        frame 3 {
          # "laser1 and laser2 are active"
          n196 = Index Array(array=w519, index #1=w497, index #2=w496, index #3=w495, index #4=w494, index #5=w493, index #6=w492, index #7=w491, index #8=w490, index #9=w489, index #10=w488, index #11=w487, index #12=w486) -> (element #1=w518:u16, element #2=w517:u16, element #3=w516:u16, element #4=w515:u16, element #5=w514:u16, element #6=w513:u16, element #7=w508:u16, element #9=w509:u16, element #10=w510:u16, element #11=w511:u16, element #12=w512:u16)  [unwired: 1 out]
          n197 = call "BRig_RT__Case_Exp__State_initTrial__LC.vi"("input_L_OnOff"=w518, "input_L_Block"=w517, "input_L_Count"=w516, "input_L_Prob"=w515, "input_L_Tdelay"=w514, "input_L_delayOpt"=w513, "input_T_state"=w507, "input_iSpout"=w483, "input_iTrial_relative"=w506, "input_L_T"=w485) -> ("output_LC_Event"=w505:bool, "output_LC_Laser"=w504:bool, "output_L_Tstart"=w503:u16, "output_L_Tend"=w502:u16)  [unwired: 6 in]
          n198 = call "BRig_RT__Case_Exp__State_initTrial__LC.vi"("input_L_OnOff"=w508, "input_L_Block"=w483, "input_L_Count"=w509, "input_L_Prob"=w510, "input_L_Tdelay"=w511, "input_L_delayOpt"=w512, "input_T_state"=w507, "input_iSpout"=w483, "input_iTrial_relative"=w506, "input_L_T"=w484) -> ("output_LC_Event"=w499:bool, "output_LC_Laser"=w501:bool, "output_L_Tstart"=w500:u16, "output_L_Tend"=w498:u16)  [unwired: 6 in]
        }
      }
      n199 = case shown="1" w17 {
        tunnel: w32 -> [_ w342 w364 w400]
        tunnel: w15 -> [_ w321 w343 w365]
        tunnel: w37 -> [_ w336 w358 w389]
        tunnel: w13 -> [_ w335 w357 w388]
        tunnel: [w319 w334 w346 w387] -> w52
        tunnel: [w319 w333 w346 w386] -> w51
        tunnel: [w320 w332 w345 w385] -> w47
        tunnel: [w320 w331 w345 w384] -> w45
        tunnel: [w319 w324 w356 w383] -> w49
        tunnel: [w320 w323 w355 w382] -> w43
        tunnel: [w319 w324 w354 w381] -> w50
        tunnel: [w320 w323 w353 w380] -> w41
        tunnel: w64 -> [_ w330 _ w379]
        tunnel: w63 -> [_ w329 _ w378]
        tunnel: w62 -> [_ w328 _ w377]
        tunnel: w61 -> [_ w327 _ w376]
        tunnel: w60 -> [_ w326 _ w375]
        tunnel: w59 -> [_ w325 _ w374]
        tunnel: w58 -> [_ _ w352 w373]
        tunnel: w57 -> [_ _ w351 w372]
        tunnel: w56 -> [_ _ w350 w371]
        tunnel: w55 -> [_ _ w349 w370]
        tunnel: w54 -> [_ _ w348 w369]
        tunnel: w53 -> [_ _ w347 w368]
        tunnel: w66 -> [_ w322 _ w367]
        tunnel: w65 -> [_ _ w344 w366]
        frame 0, Default {
          w320 = u16 0
          w319 = FALSE
          # "No active lasers"
        }
        frame 1 {
          w323 = u16 0
          w324 = FALSE
          # "laser1 is active"
          n200 = Index Array(array=w342, index #1=w330, index #2=w329, index #3=w328, index #4=w327, index #5=w326, index #6=w325) -> (element #1=w341:u16, element #3=w340:u16, element #4=w339:u16, element #5=w338:u16, element #6=w337:u16)  [unwired: 1 out]
          n201 = call "BRig_RT__Case_Exp__State_initTrial__LC.vi"("input_L_OnOff"=w341, "input_L_Block"=w321, "input_L_Count"=w340, "input_L_Prob"=w339, "input_L_Tdelay"=w338, "input_L_delayOpt"=w337, "input_T_state"=w336, "input_iSpout"=w321, "input_iTrial_relative"=w335, "input_L_T"=w322) -> ("output_LC_Event"=w334:bool, "output_LC_Laser"=w333:bool, "output_L_Tstart"=w332:u16, "output_L_Tend"=w331:u16)  [unwired: 6 in]
        }
        frame 2 {
          w345 = u16 0
          w346 = FALSE
          # "laser2 is active"
          n202 = Index Array(array=w364, index #1=w352, index #2=w351, index #3=w350, index #4=w349, index #5=w348, index #6=w347) -> (element #1=w359:u16, element #3=w360:u16, element #4=w361:u16, element #5=w362:u16, element #6=w363:u16)  [unwired: 1 out]
          n203 = call "BRig_RT__Case_Exp__State_initTrial__LC.vi"("input_L_OnOff"=w359, "input_L_Block"=w343, "input_L_Count"=w360, "input_L_Prob"=w361, "input_L_Tdelay"=w362, "input_L_delayOpt"=w363, "input_T_state"=w358, "input_iSpout"=w343, "input_iTrial_relative"=w357, "input_L_T"=w344) -> ("output_LC_Event"=w354:bool, "output_LC_Laser"=w356:bool, "output_L_Tstart"=w355:u16, "output_L_Tend"=w353:u16)  [unwired: 6 in]
        }
        frame 3 {
          # "laser1 and laser2 are active"
          n204 = Index Array(array=w400, index #1=w379, index #2=w378, index #3=w377, index #4=w376, index #5=w375, index #6=w374, index #7=w373, index #8=w372, index #9=w371, index #10=w370, index #11=w369, index #12=w368) -> (element #1=w399:u16, element #3=w398:u16, element #4=w397:u16, element #5=w396:u16, element #6=w395:u16, element #7=w390:u16, element #9=w391:u16, element #10=w392:u16, element #11=w393:u16, element #12=w394:u16)  [unwired: 2 out]
          n205 = call "BRig_RT__Case_Exp__State_initTrial__LC.vi"("input_L_OnOff"=w399, "input_L_Block"=w365, "input_L_Count"=w398, "input_L_Prob"=w397, "input_L_Tdelay"=w396, "input_L_delayOpt"=w395, "input_T_state"=w389, "input_iSpout"=w365, "input_iTrial_relative"=w388, "input_L_T"=w367) -> ("output_LC_Event"=w387:bool, "output_LC_Laser"=w386:bool, "output_L_Tstart"=w385:u16, "output_L_Tend"=w384:u16)  [unwired: 6 in]
          n206 = call "BRig_RT__Case_Exp__State_initTrial__LC.vi"("input_L_OnOff"=w390, "input_L_Block"=w365, "input_L_Count"=w391, "input_L_Prob"=w392, "input_L_Tdelay"=w393, "input_L_delayOpt"=w394, "input_T_state"=w389, "input_iSpout"=w365, "input_iTrial_relative"=w388, "input_L_T"=w366) -> ("output_LC_Event"=w381:bool, "output_LC_Laser"=w383:bool, "output_L_Tstart"=w382:u16, "output_L_Tend"=w380:u16)  [unwired: 6 in]
        }
      }
      n207 = call "BRig_dataCurrent_L_ENL_T_start_l1.vi"() -> ("output_L_ENL_T_start_l1"=w110:i32)  [unwired: 11 in]
      n208 = call "BRig_dataCurrent_L_ENL_T_end_l1.vi"() -> ("output_L_ENL_T_end_l1"=w108:i32)  [unwired: 11 in]
      n209 = call "BRig_dataCurrent_L_ENL_T_start_l2.vi"() -> ("output_L_T_ENL1_start_l2"=w106:i32)  [unwired: 11 in]
      n210 = call "BRig_dataCurrent_L_ENL_T_end_l2.vi"() -> ("output_L_ENL_T_end_l2"=w104:i32)  [unwired: 11 in]
      n211 = call "BRig_dataCurrent_L_ENL2_T_start_l1.vi"() -> ("output_L_ENL2_T_start_l1"=w48:i32)  [unwired: 11 in]
      n212 = call "BRig_dataCurrent_L_ENL2_T_end_l1.vi"() -> ("output_L_ENL2_T_end_l1"=w46:i32)  [unwired: 11 in]
      n213 = call "BRig_dataCurrent_L_ENL2_T_start_l2.vi"() -> ("output_L_T_ENL2_start_l2"=w44:i32)  [unwired: 11 in]
      n214 = call "BRig_dataCurrent_L_ENL2_T_end_l2.vi"() -> ("output_L_ENL2_T_end_l2"=w42:i32)  [unwired: 11 in]
      n215 = Replace Array Subset(array=w112, new element #1=w109, index #1=w110, new element #2=w107, index #2=w108, new element #3=w105, index #3=w106, new element #4=w103, index #4=w104, new element #5=w47, index #5=w48, new element #6=w45, index #6=w46, new element #7=w43, index #7=w44, new element #8=w41, index #8=w42) -> (w111:u16[])
      n216 = call "BRig_dataTrial_L_ENL_event_I_l1.vi"() -> ("output_L_ENL_event_I_l1"=w125:i32)  [unwired: 11 in]
      n217 = call "BRig_dataTrial_L_ENL_trig_I_l1.vi"() -> ("output_L_ENL_trig_I_l1"=w122:i32)  [unwired: 11 in]
      n218 = call "BRig_dataTrial_L_ENL_event_I_l2.vi"() -> ("output_L_ENL_event_I_l2"=w121:i32)  [unwired: 11 in]
      n219 = call "BRig_dataTrial_L_ENL_trig_I_l2.vi"() -> ("output_L_ENL_trig_I_l2"=w120:i32)  [unwired: 11 in]
      n220 = call "BRig_dataTrial_L_ENL2_event_I_l1.vi"() -> ("output_L_ENL2_event_I_l1"=w75:i32)  [unwired: 11 in]
      n221 = call "BRig_dataTrial_L_ENL2_trig_I_l1.vi"() -> ("output_L_ENL2_trig_I_l1"=w74:i32)  [unwired: 11 in]
      n222 = call "BRig_dataTrial_L_ENL2_event_I_l2.vi"() -> ("output_L_ENL2_event_I_l2"=w73:i32)  [unwired: 11 in]
      n223 = call "BRig_dataTrial_L_ENL2_trig_I_l2.vi"() -> ("output_L_ENL2_trig_I_l2"=w71:i32)  [unwired: 11 in]
      n224 = call "BRig_arrTrig_L_ENL_event_l1.vi"() -> ("output_L_ENL_event_l1"=w133:i32)  [unwired: 11 in]
      n225 = call "BRig_arrTrig_L_ENL_laser_l1.vi"() -> ("output_L_ENL_laserTrig_l1"=w132:i32)  [unwired: 11 in]
      n226 = call "BRig_arrTrig_L_ENL_event_l2.vi"() -> ("output_L_ENL_event_l2"=w131:i32)  [unwired: 11 in]
      n227 = call "BRig_arrTrig_L_ENL_laser_l2.vi"() -> ("output_L_ENL_laserTrig_l2"=w130:i32)  [unwired: 11 in]
      n228 = call "BRig_arrTrig_L_ENL2_event_l1.vi"() -> ("output_L_ENL2_event_l1"=w83:i32)  [unwired: 11 in]
      n229 = call "BRig_arrTrig_L_ENL2_laser_l1.vi"() -> ("output_L_ENL2_laserTrig_l1"=w82:i32)  [unwired: 11 in]
      n230 = call "BRig_arrTrig_L_ENL2_event_l2.vi"() -> ("output_L_ENL2_event_l2"=w81:i32)  [unwired: 11 in]
      n231 = call "BRig_arrTrig_L_ENL2_laser_l2.vi"() -> ("output_L_ENL2_laserTrig_l2"=w80:i32)  [unwired: 11 in]
      n232 = Boolean To (0,1)(Boolean=w124) -> (0, 1=w129:i16)
      n233 = Boolean To (0,1)(Boolean=w118) -> (0, 1=w128:i16)
      n234 = Boolean To (0,1)(Boolean=w116) -> (0, 1=w126:i16)
      n235 = Boolean To (0,1)(Boolean=w114) -> (0, 1=w127:i16)
      n236 = Boolean To (0,1)(Boolean=w52) -> (0, 1=w79:i16)
      n237 = Boolean To (0,1)(Boolean=w51) -> (0, 1=w78:i16)
      n238 = Boolean To (0,1)(Boolean=w50) -> (0, 1=w76:i16)
      n239 = Boolean To (0,1)(Boolean=w49) -> (0, 1=w77:i16)
      n240 = Replace Array Subset(array=w135, new element #1=w124, index #1=w133, new element #2=w118, index #2=w132, new element #3=w116, index #3=w131, new element #4=w114, index #4=w130, new element #5=w52, index #5=w83, new element #6=w51, index #6=w82, new element #7=w50, index #7=w81, new element #8=w49, index #8=w80) -> (w134:bool[])
      n241 = To Unsigned Word Integer(number=w129) -> (unsigned 16bit integer=w123:u16)
      n242 = To Unsigned Word Integer(number=w128) -> (unsigned 16bit integer=w119:u16)
      n243 = To Unsigned Word Integer(number=w126) -> (unsigned 16bit integer=w117:u16)
      n244 = To Unsigned Word Integer(number=w127) -> (unsigned 16bit integer=w115:u16)
      n245 = To Unsigned Word Integer(number=w79) -> (unsigned 16bit integer=w70:u16)
      n246 = To Unsigned Word Integer(number=w78) -> (unsigned 16bit integer=w69:u16)
      n247 = To Unsigned Word Integer(number=w76) -> (unsigned 16bit integer=w68:u16)
      n248 = To Unsigned Word Integer(number=w77) -> (unsigned 16bit integer=w67:u16)
      n249 = Replace Array Subset(array=w34, new element #1=w123, index (row) #1=w72, index (col) #1=w125, new element #2=w119, index (row) #2=w72, index (col) #2=w122, new element #3=w117, index (row) #3=w72, index (col) #3=w121, new element #4=w115, index (row) #4=w72, index (col) #4=w120, new element #5=w70, index (row) #5=w72, index (col) #5=w75, new element #6=w69, index (row) #6=w72, index (col) #6=w74, new element #7=w68, index (row) #7=w72, index (col) #7=w73, new element #8=w67, index (row) #8=w72, index (col) #8=w71) -> (w113:u16[][])
    }
    frame False {
      w580 = 0
      # "Record laser timing"
      # "Calculate laser timing"
      # "Total Time (ENL2)"
      # "Total Time (ENL)"
      # "iTrial\nrelative"
      # "Total Time (Laser 2)"
      # "Total Time (Laser 1)"
      # "Current directionality, L or R?"
      # "laser timing case (ENL2)"
      # "Determine case for\ncalculating laser timing"
      # "2) Get relative iTrial"
      # "1) If Trial Start State = PostReward,\nThen check LC_ENL_nReward"
      # "laser2 active (ENL2)?"
      # "laser1 active (ENL2)?"
      # "laser2 active (ENL)?"
      # "laser1 active (ENL)?"
      # "1) If Trial Start State = PostReward,\nThen check LC_ENL_nReward\n\n2) Get relative iTrial"
      # "Gather variables"
      # "Last trial's\niReward\n(0 = not reward)"
      # "nTrials, current block"
      # "idx dataTrial"
      # "Total Time (ENL2)"
      # "Total Time (ENL)"
      # "# PostReward Trials"
      # "Current directionality, L or R?"
      # "Have ENL2?"
      # "Total Time (Laser 2)"
      # "Total Time (Laser 1)"
      # "Calculate settings for ENL2"
      # "Calculate settings for ENL"
      # "Set laser settings for ENL and ENL2"
      # "iTrial\nrelative"
      # "laser timing case (ENL)"
      # "Trial start state\n0 (unknown)\n1 (first)\n2 (PreReward)\n3 (PostReward)"
      # "laser2 active?"
      # "laser1 active?"
      n250 = call "BRig_dataCurrent_iSpout.vi"() -> ("output_iSpout"=w644:i32)  [unwired: 11 in]
      n251 = call "BRig_dataCurrent_LaserSwitch_l1.vi"() -> ("output_LaserSwitch_l1"=w653:i32)  [unwired: 11 in]
      n252 = call "BRig_dataCurrent_LaserSwitch_l2.vi"() -> ("output_LaserSwitch_l2"=w652:i32)  [unwired: 11 in]
      n253 = call "BRig_dataCurrent_iTrial.vi"() -> ("output_iTrial"=w593:i32)  [unwired: 11 in]
      n254 = call "BRig_dataExp_L_Ttotal_l1.vi"() -> ("output_L_Ttotal_l1"=w597:i32)  [unwired: 11 in]
      n255 = call "BRig_dataExp_L_Ttotal_l2.vi"() -> ("output_L_Ttotal_l2"=w598:i32)  [unwired: 11 in]
      n256 = call "BRig_dataExp_I_Cue2.vi"() -> ("output_I_Cue2"=w547:i32)  [unwired: 11 in]
      n257 = call "BRig_dataTrial_sTrial_start.vi"() -> ("output_sTrial_start"=w649:i32)  [unwired: 11 in]
      n258 = call "BRig_dataTrial_iTrial_PostR.vi"() -> ("output_iTrial_PostR"=w594:i32)  [unwired: 11 in]
      n259 = call "BRig_dataTrial_T_ENL.vi"() -> ("output_T_ENL"=w595:i32)  [unwired: 11 in]
      n260 = call "BRig_dataTrial_T_ENL2.vi"() -> ("output_T_ENL2"=w592:i32)  [unwired: 11 in]
      n261 = Index Array(array=w620, index #1=w644, index #2=w653, index #3=w652, index #4=w593) -> (element #1=w572:u16, element #2=w651:u16, element #3=w650:u16, element #4=w533:u16)
      n262 = Index Array(array=w596, index #1=w597, index #2=w598, index #3=w547) -> (element #1=w574:u16, element #2=w573:u16, element #3=w546:u16)
      n263 = Index Array(array=w541, index (row) #1=w580, index (col) #1=w649, index (row) #2=w580, index (col) #2=w594, index (row) #3=w580, index (col) #3=w595, index (row) #4=w580, index (col) #4=w592) -> (element #1=w531:u16, element #2=w532:u16, element #3=w545:u16, element #4=w544:u16)
      n264 = Not Equal To 0?(x=w546) -> (x != 0?=w536:bool)
      n265 = call "BRig_dataTrial_iReward.vi"() -> ("output_iReward"=w542:i32)  [unwired: 11 in]
      n266 = Not Equal To 0?(x=w651) -> (x != 0?=w537:bool)
      n267 = Not Equal To 0?(x=w650) -> (x != 0?=w538:bool)
      n268 = Index Array(array=w541, index (row)=1 ("disabled index (row)"), index (col)=w542) -> (element=w540:u16)
      n269 = case shown="3" w531 {
        tunnel: w540 -> [_ _ w668]
        tunnel: w539 -> [_ _ w669]
        tunnel: w538 -> [_ w658 w661]
        tunnel: w537 -> [_ w659 w662]
        tunnel: w536 -> [_ w657 w660]
        tunnel: [w654 w659 w667] -> w529
        tunnel: [w654 w658 w666] -> w528
        tunnel: [w654 w656 w665] -> w523
        tunnel: [w654 w655 w664] -> w522
        frame 0 {
          w654 = FALSE
        }
        frame 1, Default {
          n270 = And(x=w657, y=w659) -> (x .and. y?=w656:bool)
          n271 = And(x=w658, y=w657) -> (x .and. y?=w655:bool)
        }
        frame 3 {
          w674 = i16 0 ("f")
          n272 = Boolean To (0,1)(Boolean=w662) -> (0, 1=w672:i16)
          n273 = Select(t=i16 2, s=w661, f=w674) -> (s? t:f=w673:i16)
          n274 = Select(t=i16 4, s=w660, f=w674) -> (s? t:f=w671:i16)
          n275 = Compound Arithmetic op=ADD(w672, w673, w671) -> (w670:i16)
          n276 = case shown="7" w670 {
            tunnel: w669 -> [_ w681 w692 w704 _ w731 w754 w777]
            tunnel: w668 -> [_ w680 w691 w703 _ w727 w750 w762]
            tunnel: [w677 w679 w689 w702 w719 w726 w747 w761] -> w667
            tunnel: [w677 w678 w690 w701 w719 w724 w749 w760] -> w666
            tunnel: [w677 w678 w689 w700 w719 w725 w747 w759] -> w665
            tunnel: [w677 w678 w689 w700 w719 w724 w748 w758] -> w664
            tunnel: FALSE -> [w677 w678 w689 w700 w719 w724 w747 _]
            frame 0, Default {
            }
            frame 1 {
              n277 = call "BRig_dataLC_ENL_PostR_nRew1_l1.vi"() -> ("output_ENL_PostR_nRew1_l1"=w688:i32)  [unwired: 11 in]
              n278 = call "BRig_dataLC_ENL_PostR_nRew2_l1.vi"() -> ("output_ENL_PostR_nRew2_l1"=w687:i32)  [unwired: 11 in]
              n279 = Index Array(array=w681, index #1=w688, index #2=w687) -> (element #1=w683:u16, element #2=w682:u16)
              n280 = Equal To 0?(x=w683) -> (x = 0?=w684:bool)
              n281 = Equal?(x=w683, y=w680) -> (x = y?=w685:bool)
              n282 = Equal?(x=w682, y=w680) -> (x = y?=w686:bool)
              n283 = Compound Arithmetic op=OR(w684, w685, w686) -> (w679:bool)
            }
            frame 2 {
              n284 = call "BRig_dataLC_ENL_PostR_nRew1_l2.vi"() -> ("output_ENL_PostR_nRew1_l2"=w699:i32)  [unwired: 11 in]
              n285 = call "BRig_dataLC_ENL_PostR_nRew2_l2.vi"() -> ("output_ENL_PostR_nRew2_l2"=w698:i32)  [unwired: 11 in]
              n286 = Index Array(array=w692, index #1=w699, index #2=w698) -> (element #1=w693:u16, element #2=w694:u16)
              n287 = Equal To 0?(x=w693) -> (x = 0?=w696:bool)
              n288 = Equal?(x=w693, y=w691) -> (x = y?=w695:bool)
              n289 = Equal?(x=w694, y=w691) -> (x = y?=w697:bool)
              n290 = Compound Arithmetic op=OR(w696, w695, w697) -> (w690:bool)
            }
            frame 3 {
              n291 = call "BRig_dataLC_ENL_PostR_nRew1_l1.vi"() -> ("output_ENL_PostR_nRew1_l1"=w718:i32)  [unwired: 11 in]
              n292 = call "BRig_dataLC_ENL_PostR_nRew2_l1.vi"() -> ("output_ENL_PostR_nRew2_l1"=w717:i32)  [unwired: 11 in]
              n293 = call "BRig_dataLC_ENL_PostR_nRew1_l2.vi"() -> ("output_ENL_PostR_nRew1_l2"=w716:i32)  [unwired: 11 in]
              n294 = call "BRig_dataLC_ENL_PostR_nRew2_l2.vi"() -> ("output_ENL_PostR_nRew2_l2"=w715:i32)  [unwired: 11 in]
              n295 = Index Array(array=w704, index #1=w718, index #2=w717, index #3=w716, index #4=w715) -> (element #1=w708:u16, element #2=w707:u16, element #3=w705:u16, element #4=w706:u16)
              n296 = Equal To 0?(x=w708) -> (x = 0?=w709:bool)
              n297 = Equal?(x=w708, y=w703) -> (x = y?=w710:bool)
              n298 = Equal?(x=w707, y=w703) -> (x = y?=w711:bool)
              n299 = Equal To 0?(x=w705) -> (x = 0?=w713:bool)
              n300 = Equal?(x=w705, y=w703) -> (x = y?=w712:bool)
              n301 = Equal?(x=w706, y=w703) -> (x = y?=w714:bool)
              n302 = Compound Arithmetic op=OR(w709, w710, w711) -> (w702:bool)
              n303 = Compound Arithmetic op=OR(w713, w712, w714) -> (w701:bool)
            }
            frame 4 {
            }
            frame 5 {
              n304 = call "BRig_dataLC_ENL_PostR_nRew1_l1.vi"() -> ("output_ENL_PostR_nRew1_l1"=w738:i32)  [unwired: 11 in]
              n305 = call "BRig_dataLC_ENL_PostR_nRew2_l1.vi"() -> ("output_ENL_PostR_nRew2_l1"=w737:i32)  [unwired: 11 in]
              n306 = call "BRig_dataLC_ENL2_PostR_nRew1_l1.vi"() -> ("output_ENL2_PostR_nRew1_l1"=w723:i32)  [unwired: 11 in]
              n307 = call "BRig_dataLC_ENL2_PostR_nRew2_l1.vi"() -> ("output_ENL2_PostR_nRew2_l1"=w722:i32)  [unwired: 11 in]
              n308 = Index Array(array=w731, index #1=w738, index #2=w737, index #3=w723, index #4=w722) -> (element #1=w733:u16, element #2=w732:u16, element #3=w721:u16, element #4=w720:u16)
              n309 = Equal To 0?(x=w733) -> (x = 0?=w734:bool)
              n310 = Equal?(x=w733, y=w727) -> (x = y?=w735:bool)
              n311 = Equal?(x=w732, y=w727) -> (x = y?=w736:bool)
              n312 = Equal To 0?(x=w721) -> (x = 0?=w730:bool)
              n313 = Equal?(x=w721, y=w727) -> (x = y?=w729:bool)
              n314 = Equal?(x=w720, y=w727) -> (x = y?=w728:bool)
              n315 = Compound Arithmetic op=OR(w734, w735, w736) -> (w726:bool)
              n316 = Compound Arithmetic op=OR(w730, w729, w728) -> (w725:bool)
            }
            frame 6 {
              n317 = call "BRig_dataLC_ENL_PostR_nRew1_l2.vi"() -> ("output_ENL_PostR_nRew1_l2"=w746:i32)  [unwired: 11 in]
              n318 = call "BRig_dataLC_ENL_PostR_nRew2_l2.vi"() -> ("output_ENL_PostR_nRew2_l2"=w745:i32)  [unwired: 11 in]
              n319 = call "BRig_dataLC_ENL2_PostR_nRew1_l2.vi"() -> ("output_ENL2_PostR_nRew1_l2"=w742:i32)  [unwired: 11 in]
              n320 = call "BRig_dataLC_ENL2_PostR_nRew2_l2.vi"() -> ("output_ENL2_PostR_nRew2_l2"=w741:i32)  [unwired: 11 in]
              n321 = Index Array(array=w754, index #1=w746, index #2=w745, index #3=w742, index #4=w741) -> (element #1=w744:u16, element #2=w743:u16, element #3=w740:u16, element #4=w739:u16)
              n322 = Equal To 0?(x=w744) -> (x = 0?=w756:bool)
              n323 = Equal?(x=w744, y=w750) -> (x = y?=w755:bool)
              n324 = Equal?(x=w743, y=w750) -> (x = y?=w757:bool)
              n325 = Equal To 0?(x=w740) -> (x = 0?=w752:bool)
              n326 = Equal?(x=w740, y=w750) -> (x = y?=w753:bool)
              n327 = Equal?(x=w739, y=w750) -> (x = y?=w751:bool)
              n328 = Compound Arithmetic op=OR(w756, w755, w757) -> (w749:bool)
              n329 = Compound Arithmetic op=OR(w752, w753, w751) -> (w748:bool)
            }
            frame 7 {
              n330 = call "BRig_dataLC_ENL_PostR_nRew1_l1.vi"() -> ("output_ENL_PostR_nRew1_l1"=w791:i32)  [unwired: 11 in]
              n331 = call "BRig_dataLC_ENL_PostR_nRew2_l1.vi"() -> ("output_ENL_PostR_nRew2_l1"=w790:i32)  [unwired: 11 in]
              n332 = call "BRig_dataLC_ENL_PostR_nRew1_l2.vi"() -> ("output_ENL_PostR_nRew1_l2"=w789:i32)  [unwired: 11 in]
              n333 = call "BRig_dataLC_ENL_PostR_nRew2_l2.vi"() -> ("output_ENL_PostR_nRew2_l2"=w788:i32)  [unwired: 11 in]
              n334 = call "BRig_dataLC_ENL2_PostR_nRew1_l1.vi"() -> ("output_ENL2_PostR_nRew1_l1"=w776:i32)  [unwired: 11 in]
              n335 = call "BRig_dataLC_ENL2_PostR_nRew2_l1.vi"() -> ("output_ENL2_PostR_nRew2_l1"=w775:i32)  [unwired: 11 in]
              n336 = call "BRig_dataLC_ENL2_PostR_nRew1_l2.vi"() -> ("output_ENL2_PostR_nRew1_l2"=w774:i32)  [unwired: 11 in]
              n337 = call "BRig_dataLC_ENL2_PostR_nRew2_l2.vi"() -> ("output_ENL2_PostR_nRew2_l2"=w773:i32)  [unwired: 11 in]
              n338 = Index Array(array=w777, index #1=w791, index #2=w790, index #3=w789, index #4=w788, index #5=w776, index #6=w775, index #7=w774, index #8=w773) -> (element #1=w781:u16, element #2=w780:u16, element #3=w778:u16, element #4=w779:u16, element #5=w766:u16, element #6=w765:u16, element #7=w763:u16, element #8=w764:u16)
              n339 = Equal To 0?(x=w781) -> (x = 0?=w782:bool)
              n340 = Equal?(x=w781, y=w762) -> (x = y?=w783:bool)
              n341 = Equal?(x=w780, y=w762) -> (x = y?=w784:bool)
              n342 = Equal To 0?(x=w778) -> (x = 0?=w786:bool)
              n343 = Equal?(x=w778, y=w762) -> (x = y?=w785:bool)
              n344 = Equal?(x=w779, y=w762) -> (x = y?=w787:bool)
              n345 = Equal To 0?(x=w766) -> (x = 0?=w772:bool)
              n346 = Equal?(x=w766, y=w762) -> (x = y?=w771:bool)
              n347 = Equal?(x=w765, y=w762) -> (x = y?=w770:bool)
              n348 = Equal To 0?(x=w763) -> (x = 0?=w768:bool)
              n349 = Equal?(x=w763, y=w762) -> (x = y?=w769:bool)
              n350 = Equal?(x=w764, y=w762) -> (x = y?=w767:bool)
              n351 = Compound Arithmetic op=OR(w782, w783, w784) -> (w761:bool)
              n352 = Compound Arithmetic op=OR(w786, w785, w787) -> (w760:bool)
              n353 = Compound Arithmetic op=OR(w772, w771, w770) -> (w759:bool)
              n354 = Compound Arithmetic op=OR(w768, w769, w767) -> (w758:bool)
            }
          }
        }
      }
      n355 = case shown="3" w531 {
        tunnel: [w931 w943 w955] -> w610
        tunnel: [w930 w942 w944] -> w609
        tunnel: [w929 w941 w945] -> w608
        tunnel: [w928 w940 w946] -> w607
        tunnel: [w927 w939 w947] -> w606
        tunnel: [w926 w938 w948] -> w605
        tunnel: [w925 w937 w954] -> w604
        tunnel: [w924 w936 w953] -> w603
        tunnel: [w923 w935 w952] -> w602
        tunnel: [w922 w934 w951] -> w601
        tunnel: [w921 w933 w950] -> w600
        tunnel: [w920 w932 w949] -> w599
        frame 1, Default {
          n356 = call "BRig_dataLC_ENL_First_OnOff_l1.vi"() -> ("output_ENL_First_OnOff"=w931:i32)  [unwired: 11 in]
          n357 = call "BRig_dataLC_ENL_First_Block_l1.vi"() -> ("output_ENL_First_Block"=w930:i32)  [unwired: 11 in]
          n358 = call "BRig_dataLC_ENL_First_Count_l1.vi"() -> ("output_ENL_First_Count"=w929:i32)  [unwired: 11 in]
          n359 = call "BRig_dataLC_ENL_First_Prob_l1.vi"() -> ("output_ENL_First_Prob"=w928:i32)  [unwired: 11 in]
          n360 = call "BRig_dataLC_ENL_First_Delay_l1.vi"() -> ("output_ENL_First_Delay"=w927:i32)  [unwired: 11 in]
          n361 = call "BRig_dataLC_ENL_First_DelayOpt_l1.vi"() -> ("output_ENL_First_DelayOpt"=w926:i32)  [unwired: 11 in]
          n362 = call "BRig_dataLC_ENL_First_OnOff_l2.vi"() -> ("output_ENL_First_OnOff_l2"=w925:i32)  [unwired: 11 in]
          n363 = call "BRig_dataLC_ENL_First_Block_l2.vi"() -> ("output_ENL_First_Block_l2"=w924:i32)  [unwired: 11 in]
          n364 = call "BRig_dataLC_ENL_First_Count_l2.vi"() -> ("output_ENL_First_Count_l2"=w923:i32)  [unwired: 11 in]
          n365 = call "BRig_dataLC_ENL_First_Prob_l2.vi"() -> ("output_ENL_First_Prob_l2"=w922:i32)  [unwired: 11 in]
          n366 = call "BRig_dataLC_ENL_First_Delay_l2.vi"() -> ("output_ENL_First_Delay_l2"=w921:i32)  [unwired: 11 in]
          n367 = call "BRig_dataLC_ENL_First_DelayOpt_l2.vi"() -> ("output_ENL_First_DelayOpt_l2"=w920:i32)  [unwired: 11 in]
        }
        frame 2 {
          n368 = call "BRig_dataLC_ENL_PreR_OnOff_l1.vi"() -> ("output_ENL_PreR_OnOff"=w943:i32)  [unwired: 11 in]
          n369 = call "BRig_dataLC_ENL_PreR_Block_l1.vi"() -> ("output_ENL_PreR_Block"=w942:i32)  [unwired: 11 in]
          n370 = call "BRig_dataLC_ENL_PreR_Count_l1.vi"() -> ("output_ENL_PreR_Count"=w941:i32)  [unwired: 11 in]
          n371 = call "BRig_dataLC_ENL_PreR_Prob_l1.vi"() -> ("output_ENL_PreR_Prob"=w940:i32)  [unwired: 11 in]
          n372 = call "BRig_dataLC_ENL_PreR_Delay_l1.vi"() -> ("output_ENL_PreR_Delay"=w939:i32)  [unwired: 11 in]
          n373 = call "BRig_dataLC_ENL_PreR_DelayOpt_l1.vi"() -> ("output_ENL_PreR_DelayOpt"=w938:i32)  [unwired: 11 in]
          n374 = call "BRig_dataLC_ENL_PreR_OnOff_l2.vi"() -> ("output_ENL_PreR_OnOff_l2"=w937:i32)  [unwired: 11 in]
          n375 = call "BRig_dataLC_ENL_PreR_Block_l2.vi"() -> ("output_ENL_PreR_Block_l2"=w936:i32)  [unwired: 11 in]
          n376 = call "BRig_dataLC_ENL_PreR_Count_l2.vi"() -> ("output_ENL_PreR_Count_l2"=w935:i32)  [unwired: 11 in]
          n377 = call "BRig_dataLC_ENL_PreR_Prob_l2.vi"() -> ("output_ENL_PreR_Prob_l2"=w934:i32)  [unwired: 11 in]
          n378 = call "BRig_dataLC_ENL_PreR_Delay_l2.vi"() -> ("output_ENL_PreR_Delay_l2"=w933:i32)  [unwired: 11 in]
          n379 = call "BRig_dataLC_ENL_PreR_DelayOpt_l2.vi"() -> ("output_ENL_PreR_DelayOpt_l2"=w932:i32)  [unwired: 11 in]
        }
        frame 3 {
          n380 = call "BRig_dataLC_ENL_PostR_OnOff_l1.vi"() -> ("output_ENL_PostR_OnOff"=w955:i32)  [unwired: 11 in]
          n381 = call "BRig_dataLC_ENL_PostR_Block_l1.vi"() -> ("output_ENL_PostR_Block"=w944:i32)  [unwired: 11 in]
          n382 = call "BRig_dataLC_ENL_PostR_Count_l1.vi"() -> ("output_ENL_PostR_Count"=w945:i32)  [unwired: 11 in]
          n383 = call "BRig_dataLC_ENL_PostR_Prob_l1.vi"() -> ("output_ENL_PostR_Prob"=w946:i32)  [unwired: 11 in]
          n384 = call "BRig_dataLC_ENL_PostR_Delay_l1.vi"() -> ("output_ENL_PostR_Delay"=w947:i32)  [unwired: 11 in]
          n385 = call "BRig_dataLC_ENL_PostR_DelayOpt_l1.vi"() -> ("output_ENL_PostR_DelayOpt"=w948:i32)  [unwired: 11 in]
          n386 = call "BRig_dataLC_ENL_PostR_OnOff_l2.vi"() -> ("output_ENL_PostR_OnOff_l2"=w954:i32)  [unwired: 11 in]
          n387 = call "BRig_dataLC_ENL_PostR_Block_l2.vi"() -> ("output_ENL_PostR_Block_l2"=w953:i32)  [unwired: 11 in]
          n388 = call "BRig_dataLC_ENL_PostR_Count_l2.vi"() -> ("output_ENL_PostR_Count_l2"=w952:i32)  [unwired: 11 in]
          n389 = call "BRig_dataLC_ENL_PostR_Prob_l2.vi"() -> ("output_ENL_PostR_Prob_l2"=w951:i32)  [unwired: 11 in]
          n390 = call "BRig_dataLC_ENL_PostR_Delay_l2.vi"() -> ("output_ENL_PostR_Delay_l2"=w950:i32)  [unwired: 11 in]
          n391 = call "BRig_dataLC_ENL_PostR_DelayOpt_l2.vi"() -> ("output_ENL_PostR_DelayOpt_l2"=w949:i32)  [unwired: 11 in]
        }
      }
      n392 = case shown="1, Default" w531 {
        tunnel: [w803 w815 w827] -> w571
        tunnel: [w802 w814 w826] -> w570
        tunnel: [w801 w813 w825] -> w569
        tunnel: [w800 w812 w824] -> w568
        tunnel: [w799 w811 w823] -> w567
        tunnel: [w798 w810 w822] -> w566
        tunnel: [w797 w809 w821] -> w565
        tunnel: [w796 w808 w820] -> w564
        tunnel: [w795 w807 w819] -> w563
        tunnel: [w794 w806 w818] -> w562
        tunnel: [w793 w805 w817] -> w561
        tunnel: [w792 w804 w816] -> w560
        frame 1, Default {
          n393 = call "BRig_dataLC_ENL2_First_OnOff_l1.vi"() -> ("output_ENL2_First_OnOff"=w803:i32)  [unwired: 11 in]
          n394 = call "BRig_dataLC_ENL2_First_Block_l1.vi"() -> ("output_ENL2_First_Block"=w802:i32)  [unwired: 11 in]
          n395 = call "BRig_dataLC_ENL2_First_Count_l1.vi"() -> ("output_ENL2_First_Count"=w801:i32)  [unwired: 11 in]
          n396 = call "BRig_dataLC_ENL2_First_Prob_l1.vi"() -> ("output_ENL2_First_Prob"=w800:i32)  [unwired: 11 in]
          n397 = call "BRig_dataLC_ENL2_First_Delay_l1.vi"() -> ("output_ENL2_First_Delay"=w799:i32)  [unwired: 11 in]
          n398 = call "BRig_dataLC_ENL2_First_DelayOpt_l1.vi"() -> ("output_ENL2_First_DelayOpt"=w798:i32)  [unwired: 11 in]
          n399 = call "BRig_dataLC_ENL2_First_OnOff_l2.vi"() -> ("output_ENL2_First_OnOff_l2"=w797:i32)  [unwired: 11 in]
          n400 = call "BRig_dataLC_ENL2_First_Block_l2.vi"() -> ("output_ENL2_First_Block_l2"=w796:i32)  [unwired: 11 in]
          n401 = call "BRig_dataLC_ENL2_First_Count_l2.vi"() -> ("output_ENL2_First_Count_l2"=w795:i32)  [unwired: 11 in]
          n402 = call "BRig_dataLC_ENL2_First_Prob_l2.vi"() -> ("output_ENL2_First_Prob_l2"=w794:i32)  [unwired: 11 in]
          n403 = call "BRig_dataLC_ENL2_First_Delay_l2.vi"() -> ("output_ENL2_First_Delay_l2"=w793:i32)  [unwired: 11 in]
          n404 = call "BRig_dataLC_ENL2_First_DelayOpt_l2.vi"() -> ("output_ENL2_First_DelayOpt_l2"=w792:i32)  [unwired: 11 in]
        }
        frame 2 {
          n405 = call "BRig_dataLC_ENL2_PreR_OnOff_l1.vi"() -> ("output_ENL2_PreR_OnOff"=w815:i32)  [unwired: 11 in]
          n406 = call "BRig_dataLC_ENL2_PreR_Block_l1.vi"() -> ("output_ENL2_PreR_Block"=w814:i32)  [unwired: 11 in]
          n407 = call "BRig_dataLC_ENL2_PreR_Count_l1.vi"() -> ("output_ENL2_PreR_Count"=w813:i32)  [unwired: 11 in]
          n408 = call "BRig_dataLC_ENL2_PreR_Prob_l1.vi"() -> ("output_ENL2_PreR_Prob"=w812:i32)  [unwired: 11 in]
          n409 = call "BRig_dataLC_ENL2_PreR_Delay_l1.vi"() -> ("output_ENL2_PreR_Delay"=w811:i32)  [unwired: 11 in]
          n410 = call "BRig_dataLC_ENL2_PreR_DelayOpt_l1.vi"() -> ("output_ENL2_PreR_DelayOpt"=w810:i32)  [unwired: 11 in]
          n411 = call "BRig_dataLC_ENL2_PreR_OnOff_l2.vi"() -> ("output_ENL2_PreR_OnOff_l2"=w809:i32)  [unwired: 11 in]
          n412 = call "BRig_dataLC_ENL2_PreR_Block_l2.vi"() -> ("output_ENL2_PreR_Block_l2"=w808:i32)  [unwired: 11 in]
          n413 = call "BRig_dataLC_ENL2_PreR_Count_l2.vi"() -> ("output_ENL2_PreR_Count_l2"=w807:i32)  [unwired: 11 in]
          n414 = call "BRig_dataLC_ENL2_PreR_Prob_l2.vi"() -> ("output_ENL2_PreR_Prob_l2"=w806:i32)  [unwired: 11 in]
          n415 = call "BRig_dataLC_ENL2_PreR_Delay_l2.vi"() -> ("output_ENL2_PreR_Delay_l2"=w805:i32)  [unwired: 11 in]
          n416 = call "BRig_dataLC_ENL2_PreR_DelayOpt_l2.vi"() -> ("output_ENL2_PreR_DelayOpt_l2"=w804:i32)  [unwired: 11 in]
        }
        frame 3 {
          n417 = call "BRig_dataLC_ENL2_PostR_OnOff_l1.vi"() -> ("output_ENL2_PostR_OnOff"=w827:i32)  [unwired: 11 in]
          n418 = call "BRig_dataLC_ENL2_PostR_Block_l1.vi"() -> ("output_ENL2_PostR_Block"=w826:i32)  [unwired: 11 in]
          n419 = call "BRig_dataLC_ENL2_PostR_Count_l1.vi"() -> ("output_ENL2_PostR_Count"=w825:i32)  [unwired: 11 in]
          n420 = call "BRig_dataLC_ENL2_PostR_Prob_l1.vi"() -> ("output_ENL2_PostR_Prob"=w824:i32)  [unwired: 11 in]
          n421 = call "BRig_dataLC_ENL2_PostR_Delay_l1.vi"() -> ("output_ENL2_PostR_Delay"=w823:i32)  [unwired: 11 in]
          n422 = call "BRig_dataLC_ENL2_PostR_DelayOpt_l1.vi"() -> ("output_ENL2_PostR_DelayOpt"=w822:i32)  [unwired: 11 in]
          n423 = call "BRig_dataLC_ENL2_PostR_OnOff_l2.vi"() -> ("output_ENL2_PostR_OnOff_l2"=w821:i32)  [unwired: 11 in]
          n424 = call "BRig_dataLC_ENL2_PostR_Block_l2.vi"() -> ("output_ENL2_PostR_Block_l2"=w820:i32)  [unwired: 11 in]
          n425 = call "BRig_dataLC_ENL2_PostR_Count_l2.vi"() -> ("output_ENL2_PostR_Count_l2"=w819:i32)  [unwired: 11 in]
          n426 = call "BRig_dataLC_ENL2_PostR_Prob_l2.vi"() -> ("output_ENL2_PostR_Prob_l2"=w818:i32)  [unwired: 11 in]
          n427 = call "BRig_dataLC_ENL2_PostR_Delay_l2.vi"() -> ("output_ENL2_PostR_Delay_l2"=w817:i32)  [unwired: 11 in]
          n428 = call "BRig_dataLC_ENL2_PostR_DelayOpt_l2.vi"() -> ("output_ENL2_PostR_DelayOpt_l2"=w816:i32)  [unwired: 11 in]
        }
      }
      n429 = Less?(x=w531, y=u16 3) -> (x < y?=w534:bool)
      n430 = Select(t=w533, s=w534, f=w532) -> (s? t:f=w530:u16)
      n431 = Boolean To (0,1)(Boolean=w529) -> (0, 1=w646:i16)
      n432 = Boolean To (0,1)(Boolean=w523) -> (0, 1=w526:i16)
      n433 = Select(t=i16 2, s=w528, f=i16 0) -> (s? t:f=w647:i16)
      n434 = Select(t=i16 2, s=w522, f=i16 0) -> (s? t:f=w525:i16)
      n435 = Add(x=w646, y=w647) -> (x+y=w521:i16)
      n436 = Add(x=w526, y=w525) -> (x+y=w520:i16)
      n437 = case shown="2" w521 {
        tunnel: w539 -> [_ w986 w1009 w1047]
        tunnel: w572 -> [_ w978 w1001 w1033]
        tunnel: w545 -> [_ w979 w1002 w1034]
        tunnel: w530 -> [_ w977 w1000 w1032]
        tunnel: [w956 w976 w989 w1031] -> w632
        tunnel: [w956 w975 w989 w1030] -> w626
        tunnel: [w957 w974 w988 w1029] -> w617
        tunnel: [w957 w973 w988 w1028] -> w615
        tunnel: [w956 w960 w999 w1027] -> w622
        tunnel: [w957 w959 w998 w1026] -> w613
        tunnel: [w956 w960 w997 w1025] -> w624
        tunnel: [w957 w959 w996 w1024] -> w611
        tunnel: w610 -> [_ w972 _ w1023]
        tunnel: w609 -> [_ w971 _ w1022]
        tunnel: w608 -> [_ w970 _ w1021]
        tunnel: w607 -> [_ w969 _ w1020]
        tunnel: w606 -> [_ w968 _ w1019]
        tunnel: w605 -> [_ w967 _ w1018]
        tunnel: w604 -> [_ w966 w995 w1017]
        tunnel: w603 -> [_ w965 w994 w1016]
        tunnel: w602 -> [_ w964 w993 w1015]
        tunnel: w601 -> [_ w963 w992 w1014]
        tunnel: w600 -> [_ w962 w991 w1013]
        tunnel: w599 -> [_ w961 w990 w1012]
        tunnel: w574 -> [_ w958 _ w1011]
        tunnel: w573 -> [_ _ w987 w1010]
        frame 0, Default {
          w957 = u16 0
          w956 = FALSE
          # "No active lasers"
        }
        frame 1 {
          w959 = u16 0
          w960 = FALSE
          # "laser1 is active"
          n438 = Index Array(array=w986, index #1=w972, index #2=w971, index #3=w970, index #4=w969, index #5=w968, index #6=w967, index #7=w966, index #8=w965, index #9=w964, index #10=w963, index #11=w962, index #12=w961) -> (element #1=w985:u16, element #2=w984:u16, element #3=w983:u16, element #4=w982:u16, element #5=w981:u16, element #6=w980:u16)  [unwired: 6 out]
          n439 = call "BRig_RT__Case_Exp__State_initTrial__LC.vi"("input_L_OnOff"=w985, "input_L_Block"=w984, "input_L_Count"=w983, "input_L_Prob"=w982, "input_L_Tdelay"=w981, "input_L_delayOpt"=w980, "input_T_state"=w979, "input_iSpout"=w978, "input_iTrial_relative"=w977, "input_L_T"=w958) -> ("output_LC_Event"=w976:bool, "output_LC_Laser"=w975:bool, "output_L_Tstart"=w974:u16, "output_L_Tend"=w973:u16)  [unwired: 6 in]
        }
        frame 2 {
          w988 = u16 0
          w989 = FALSE
          # "laser2 is active"
          n440 = Index Array(array=w1009, index #1=w995, index #2=w994, index #3=w993, index #4=w992, index #5=w991, index #6=w990) -> (element #1=w1003:u16, element #2=w1004:u16, element #3=w1005:u16, element #4=w1006:u16, element #5=w1007:u16, element #6=w1008:u16)
          n441 = call "BRig_RT__Case_Exp__State_initTrial__LC.vi"("input_L_OnOff"=w1003, "input_L_Block"=w1004, "input_L_Count"=w1005, "input_L_Prob"=w1006, "input_L_Tdelay"=w1007, "input_L_delayOpt"=w1008, "input_T_state"=w1002, "input_iSpout"=w1001, "input_iTrial_relative"=w1000, "input_L_T"=w987) -> ("output_LC_Event"=w997:bool, "output_LC_Laser"=w999:bool, "output_L_Tstart"=w998:u16, "output_L_Tend"=w996:u16)  [unwired: 6 in]
        }
        frame 3 {
          # "laser1 and laser2 are active"
          n442 = Index Array(array=w1047, index #1=w1023, index #2=w1022, index #3=w1021, index #4=w1020, index #5=w1019, index #6=w1018, index #7=w1017, index #8=w1016, index #9=w1015, index #10=w1014, index #11=w1013, index #12=w1012) -> (element #1=w1046:u16, element #2=w1045:u16, element #3=w1044:u16, element #4=w1043:u16, element #5=w1042:u16, element #6=w1041:u16, element #7=w1035:u16, element #8=w1036:u16, element #9=w1037:u16, element #10=w1038:u16, element #11=w1039:u16, element #12=w1040:u16)
          n443 = call "BRig_RT__Case_Exp__State_initTrial__LC.vi"("input_L_OnOff"=w1046, "input_L_Block"=w1045, "input_L_Count"=w1044, "input_L_Prob"=w1043, "input_L_Tdelay"=w1042, "input_L_delayOpt"=w1041, "input_T_state"=w1034, "input_iSpout"=w1033, "input_iTrial_relative"=w1032, "input_L_T"=w1011) -> ("output_LC_Event"=w1031:bool, "output_LC_Laser"=w1030:bool, "output_L_Tstart"=w1029:u16, "output_L_Tend"=w1028:u16)  [unwired: 6 in]
          n444 = call "BRig_RT__Case_Exp__State_initTrial__LC.vi"("input_L_OnOff"=w1035, "input_L_Block"=w1036, "input_L_Count"=w1037, "input_L_Prob"=w1038, "input_L_Tdelay"=w1039, "input_L_delayOpt"=w1040, "input_T_state"=w1034, "input_iSpout"=w1033, "input_iTrial_relative"=w1032, "input_L_T"=w1010) -> ("output_LC_Event"=w1025:bool, "output_LC_Laser"=w1027:bool, "output_L_Tstart"=w1026:u16, "output_L_Tend"=w1024:u16)  [unwired: 6 in]
        }
      }
      n445 = case shown="3" w520 {
        tunnel: w539 -> [_ w858 w881 w919]
        tunnel: w572 -> [_ w850 w873 w905]
        tunnel: w544 -> [_ w851 w874 w906]
        tunnel: w530 -> [_ w849 w872 w904]
        tunnel: [w828 w848 w861 w903] -> w559
        tunnel: [w828 w847 w861 w902] -> w558
        tunnel: [w829 w846 w860 w901] -> w554
        tunnel: [w829 w845 w860 w900] -> w552
        tunnel: [w828 w832 w871 w899] -> w556
        tunnel: [w829 w831 w870 w898] -> w550
        tunnel: [w828 w832 w869 w897] -> w557
        tunnel: [w829 w831 w868 w896] -> w548
        tunnel: w571 -> [_ w844 _ w895]
        tunnel: w570 -> [_ w843 _ w894]
        tunnel: w569 -> [_ w842 _ w893]
        tunnel: w568 -> [_ w841 _ w892]
        tunnel: w567 -> [_ w840 _ w891]
        tunnel: w566 -> [_ w839 _ w890]
        tunnel: w565 -> [_ w838 w867 w889]
        tunnel: w564 -> [_ w837 w866 w888]
        tunnel: w563 -> [_ w836 w865 w887]
        tunnel: w562 -> [_ w835 w864 w886]
        tunnel: w561 -> [_ w834 w863 w885]
        tunnel: w560 -> [_ w833 w862 w884]
        tunnel: w574 -> [_ w830 _ w883]
        tunnel: w573 -> [_ _ w859 w882]
        frame 0, Default {
          w829 = u16 0
          w828 = FALSE
          # "No active lasers"
        }
        frame 1 {
          w831 = u16 0
          w832 = FALSE
          # "laser1 is active"
          n446 = Index Array(array=w858, index #1=w844, index #2=w843, index #3=w842, index #4=w841, index #5=w840, index #6=w839, index #7=w838, index #8=w837, index #9=w836, index #10=w835, index #11=w834, index #12=w833) -> (element #1=w857:u16, element #2=w856:u16, element #3=w855:u16, element #4=w854:u16, element #5=w853:u16, element #6=w852:u16)  [unwired: 6 out]
          n447 = call "BRig_RT__Case_Exp__State_initTrial__LC.vi"("input_L_OnOff"=w857, "input_L_Block"=w856, "input_L_Count"=w855, "input_L_Prob"=w854, "input_L_Tdelay"=w853, "input_L_delayOpt"=w852, "input_T_state"=w851, "input_iSpout"=w850, "input_iTrial_relative"=w849, "input_L_T"=w830) -> ("output_LC_Event"=w848:bool, "output_LC_Laser"=w847:bool, "output_L_Tstart"=w846:u16, "output_L_Tend"=w845:u16)  [unwired: 6 in]
        }
        frame 2 {
          w860 = u16 0
          w861 = FALSE
          # "laser2 is active"
          n448 = Index Array(array=w881, index #1=w867, index #2=w866, index #3=w865, index #4=w864, index #5=w863, index #6=w862) -> (element #1=w875:u16, element #2=w876:u16, element #3=w877:u16, element #4=w878:u16, element #5=w879:u16, element #6=w880:u16)
          n449 = call "BRig_RT__Case_Exp__State_initTrial__LC.vi"("input_L_OnOff"=w875, "input_L_Block"=w876, "input_L_Count"=w877, "input_L_Prob"=w878, "input_L_Tdelay"=w879, "input_L_delayOpt"=w880, "input_T_state"=w874, "input_iSpout"=w873, "input_iTrial_relative"=w872, "input_L_T"=w859) -> ("output_LC_Event"=w869:bool, "output_LC_Laser"=w871:bool, "output_L_Tstart"=w870:u16, "output_L_Tend"=w868:u16)  [unwired: 6 in]
        }
        frame 3 {
          # "laser1 and laser2 are active"
          n450 = Index Array(array=w919, index #1=w895, index #2=w894, index #3=w893, index #4=w892, index #5=w891, index #6=w890, index #7=w889, index #8=w888, index #9=w887, index #10=w886, index #11=w885, index #12=w884) -> (element #1=w918:u16, element #2=w917:u16, element #3=w916:u16, element #4=w915:u16, element #5=w914:u16, element #6=w913:u16, element #7=w907:u16, element #8=w908:u16, element #9=w909:u16, element #10=w910:u16, element #11=w911:u16, element #12=w912:u16)
          n451 = call "BRig_RT__Case_Exp__State_initTrial__LC.vi"("input_L_OnOff"=w918, "input_L_Block"=w917, "input_L_Count"=w916, "input_L_Prob"=w915, "input_L_Tdelay"=w914, "input_L_delayOpt"=w913, "input_T_state"=w906, "input_iSpout"=w905, "input_iTrial_relative"=w904, "input_L_T"=w883) -> ("output_LC_Event"=w903:bool, "output_LC_Laser"=w902:bool, "output_L_Tstart"=w901:u16, "output_L_Tend"=w900:u16)  [unwired: 6 in]
          n452 = call "BRig_RT__Case_Exp__State_initTrial__LC.vi"("input_L_OnOff"=w907, "input_L_Block"=w908, "input_L_Count"=w909, "input_L_Prob"=w910, "input_L_Tdelay"=w911, "input_L_delayOpt"=w912, "input_T_state"=w906, "input_iSpout"=w905, "input_iTrial_relative"=w904, "input_L_T"=w882) -> ("output_LC_Event"=w897:bool, "output_LC_Laser"=w899:bool, "output_L_Tstart"=w898:u16, "output_L_Tend"=w896:u16)  [unwired: 6 in]
        }
      }
      n453 = call "BRig_dataCurrent_L_ENL_T_start_l1.vi"() -> ("output_L_ENL_T_start_l1"=w618:i32)  [unwired: 11 in]
      n454 = call "BRig_dataCurrent_L_ENL_T_end_l1.vi"() -> ("output_L_ENL_T_end_l1"=w616:i32)  [unwired: 11 in]
      n455 = call "BRig_dataCurrent_L_ENL_T_start_l2.vi"() -> ("output_L_T_ENL1_start_l2"=w614:i32)  [unwired: 11 in]
      n456 = call "BRig_dataCurrent_L_ENL_T_end_l2.vi"() -> ("output_L_ENL_T_end_l2"=w612:i32)  [unwired: 11 in]
      n457 = call "BRig_dataCurrent_L_ENL2_T_start_l1.vi"() -> ("output_L_ENL2_T_start_l1"=w555:i32)  [unwired: 11 in]
      n458 = call "BRig_dataCurrent_L_ENL2_T_end_l1.vi"() -> ("output_L_ENL2_T_end_l1"=w553:i32)  [unwired: 11 in]
      n459 = call "BRig_dataCurrent_L_ENL2_T_start_l2.vi"() -> ("output_L_T_ENL2_start_l2"=w551:i32)  [unwired: 11 in]
      n460 = call "BRig_dataCurrent_L_ENL2_T_end_l2.vi"() -> ("output_L_ENL2_T_end_l2"=w549:i32)  [unwired: 11 in]
      n461 = Replace Array Subset(array=w620, new element #1=w617, index #1=w618, new element #2=w615, index #2=w616, new element #3=w613, index #3=w614, new element #4=w611, index #4=w612, new element #5=w554, index #5=w555, new element #6=w552, index #6=w553, new element #7=w550, index #7=w551, new element #8=w548, index #8=w549) -> (w619:u16[])
      n462 = call "BRig_dataTrial_L_ENL_event_I_l1.vi"() -> ("output_L_ENL_event_I_l1"=w633:i32)  [unwired: 11 in]
      n463 = call "BRig_dataTrial_L_ENL_trig_I_l1.vi"() -> ("output_L_ENL_trig_I_l1"=w630:i32)  [unwired: 11 in]
      n464 = call "BRig_dataTrial_L_ENL_event_I_l2.vi"() -> ("output_L_ENL_event_I_l2"=w629:i32)  [unwired: 11 in]
      n465 = call "BRig_dataTrial_L_ENL_trig_I_l2.vi"() -> ("output_L_ENL_trig_I_l2"=w628:i32)  [unwired: 11 in]
      n466 = call "BRig_dataTrial_L_ENL2_event_I_l1.vi"() -> ("output_L_ENL2_event_I_l1"=w583:i32)  [unwired: 11 in]
      n467 = call "BRig_dataTrial_L_ENL2_trig_I_l1.vi"() -> ("output_L_ENL2_trig_I_l1"=w582:i32)  [unwired: 11 in]
      n468 = call "BRig_dataTrial_L_ENL2_event_I_l2.vi"() -> ("output_L_ENL2_event_I_l2"=w581:i32)  [unwired: 11 in]
      n469 = call "BRig_dataTrial_L_ENL2_trig_I_l2.vi"() -> ("output_L_ENL2_trig_I_l2"=w579:i32)  [unwired: 11 in]
      n470 = call "BRig_arrTrig_L_ENL_event_l1.vi"() -> ("output_L_ENL_event_l1"=w641:i32)  [unwired: 11 in]
      n471 = call "BRig_arrTrig_L_ENL_laser_l1.vi"() -> ("output_L_ENL_laserTrig_l1"=w640:i32)  [unwired: 11 in]
      n472 = call "BRig_arrTrig_L_ENL_event_l2.vi"() -> ("output_L_ENL_event_l2"=w639:i32)  [unwired: 11 in]
      n473 = call "BRig_arrTrig_L_ENL_laser_l2.vi"() -> ("output_L_ENL_laserTrig_l2"=w638:i32)  [unwired: 11 in]
      n474 = call "BRig_arrTrig_L_ENL2_event_l1.vi"() -> ("output_L_ENL2_event_l1"=w591:i32)  [unwired: 11 in]
      n475 = call "BRig_arrTrig_L_ENL2_laser_l1.vi"() -> ("output_L_ENL2_laserTrig_l1"=w590:i32)  [unwired: 11 in]
      n476 = call "BRig_arrTrig_L_ENL2_event_l2.vi"() -> ("output_L_ENL2_event_l2"=w589:i32)  [unwired: 11 in]
      n477 = call "BRig_arrTrig_L_ENL2_laser_l2.vi"() -> ("output_L_ENL2_laserTrig_l2"=w588:i32)  [unwired: 11 in]
      n478 = Boolean To (0,1)(Boolean=w632) -> (0, 1=w637:i16)
      n479 = Boolean To (0,1)(Boolean=w626) -> (0, 1=w636:i16)
      n480 = Boolean To (0,1)(Boolean=w624) -> (0, 1=w634:i16)
      n481 = Boolean To (0,1)(Boolean=w622) -> (0, 1=w635:i16)
      n482 = Boolean To (0,1)(Boolean=w559) -> (0, 1=w587:i16)
      n483 = Boolean To (0,1)(Boolean=w558) -> (0, 1=w586:i16)
      n484 = Boolean To (0,1)(Boolean=w557) -> (0, 1=w584:i16)
      n485 = Boolean To (0,1)(Boolean=w556) -> (0, 1=w585:i16)
      n486 = Replace Array Subset(array=w643, new element #1=w632, index #1=w641, new element #2=w626, index #2=w640, new element #3=w624, index #3=w639, new element #4=w622, index #4=w638, new element #5=w559, index #5=w591, new element #6=w558, index #6=w590, new element #7=w557, index #7=w589, new element #8=w556, index #8=w588) -> (w642:bool[])
      n487 = To Unsigned Word Integer(number=w637) -> (unsigned 16bit integer=w631:u16)
      n488 = To Unsigned Word Integer(number=w636) -> (unsigned 16bit integer=w627:u16)
      n489 = To Unsigned Word Integer(number=w634) -> (unsigned 16bit integer=w625:u16)
      n490 = To Unsigned Word Integer(number=w635) -> (unsigned 16bit integer=w623:u16)
      n491 = To Unsigned Word Integer(number=w587) -> (unsigned 16bit integer=w578:u16)
      n492 = To Unsigned Word Integer(number=w586) -> (unsigned 16bit integer=w577:u16)
      n493 = To Unsigned Word Integer(number=w584) -> (unsigned 16bit integer=w576:u16)
      n494 = To Unsigned Word Integer(number=w585) -> (unsigned 16bit integer=w575:u16)
      n495 = Replace Array Subset(array=w541, new element #1=w631, index (row) #1=w580, index (col) #1=w633, new element #2=w627, index (row) #2=w580, index (col) #2=w630, new element #3=w625, index (row) #3=w580, index (col) #3=w629, new element #4=w623, index (row) #4=w580, index (col) #4=w628, new element #5=w578, index (row) #5=w580, index (col) #5=w583, new element #6=w577, index (row) #6=w580, index (col) #6=w582, new element #7=w576, index (row) #7=w580, index (col) #7=w581, new element #8=w575, index (row) #8=w580, index (col) #8=w579) -> (w621:u16[][])
    }
  }
  "output_dataCurrent" <- w7
  "output_arrTrig" <- w10
  "output_dataTrial" <- w9
